vi "MegaAwesome_8_29_12d_JW.vi"() -> ()   [LabVIEW 2011]
uses:
  MegaAwesome_States.ctl
  <vilib>/Utility/file.llb/Read From Spreadsheet File (string).vi
  <vilib>/Utility/file.llb/Write To Spreadsheet File (string).vi
panel:
  out "Opj X Axis":string
  out "X Axis Display Type":string
  in  "Index-Sat":dbl=5.0
  in  "Index-Lin":dbl=5.0
  in  "IndexLog-Lin":dbl=5.0
  in  "IndexLog-Sat":dbl=5.0 caption="Num Pts"
  out "Lin Id-Log Used":dbl[](array[numeric])
  out "Lin-Vg Array-Log Used":dbl[](array[numeric])
  out "Total Width":dbl
  in  "New: Comments":string
  out "Save Array":string[][](array[string])
  out "Folder Index":i32 caption="Length"
  out "Sat Id-Used":dbl[](array[numeric])
  out "Sat Vg Array-Used":dbl[](array[numeric])
  out "Vg Array-Log-Used":dbl[](array[numeric])
  out "Sat Id-Log-Used":dbl[](array[numeric])
  out "Lin Id-Used":dbl[](array[numeric])
  out "Lin-Vg Array-Used":dbl[](array[numeric])
  out "Lin Vd":dbl
  out "Recorded Prop":T1
  out "Current State":T2
  in  "Main Tab Control":T3(tab)
  in  "Image Folder":path
  out "Image File":path=path "D:/UserData/Desktop/Jeremy/WFU/Research/Programs/VI mods/Image Not Found.png"
  in  "Transfer File":path
  out "Transfer Folder":path
  out "Fabrication Prop":T4
  in  "Transfer Plots":T5(tab)=enum."Saturation"
  in  "Lin-Trans Slider":dbl(slide) step=1.0 scale=-22.0..89.0 scale format="%#_1p"
  out "Sqrt-Lin":cluster{dbl[], dbl[]}[](graph)
  in  "Next Sqrt Lin":bool
  in  "Previous Sqrt Lin":bool
  in  "Sat-Trans Slider":dbl(slide) step=1.0 scale=-40.0..40.0 scale format="%#_1p"
  out "Sqrt-Sat":cluster{dbl[], dbl[]}[](graph)
  in  "Previous Sqrt Sat":bool
  in  "Next Sqrt Sat":bool
  out "Raw- Lin":cluster{dbl[], dbl[]}[](graph)
  out "Raw- Sat":cluster{dbl[], dbl[]}[](graph)
  in  "Log Plots":enum32{"Linear", "Saturation", "Transport"}(tab)=enum."Saturation"
  in  "Lin-Log Slider":dbl(slide) step=1.0 scale=-1.0..82.0 scale format="%#_1p"
  in  "Previous Log Lin":bool
  in  "Next Log Lin":bool
  out "Log-Lin":cluster{dbl[], dbl[]}[](graph)
  in  "Sat-Log Slider":dbl(slide) step=1.0 scale=-1.0..82.0 scale format="%#_1p"
  in  "Previous Log Sat":bool
  in  "Next Log Sat":bool
  out "Sat-Log":cluster{dbl[], dbl[]}[](graph)
  out "Transport":cluster{dbl[], dbl[]}[](graph)
  in  "Manual Controls":T6
  in  "File Controls":T7
  out "Date Recorded":string="Date Recorded" caption="Measured"
  out "Data Name:":string
  out "Image Name":string
  out "Index":string
  out "Date Created":string caption="Fabricated"
  in  "Comments:":string
  out "Rec: Length":dbl caption="Length" format="%#_3g"
  out "Rec: Width":dbl caption="Width" format="%#_4g"
  out "Rec: Dielectric (d)":dbl caption="Dielectric (d)" format="%#_3g"
  in  "New: Dielectric":dbl
  in  "New: Length":dbl
  in  "New: Width":dbl
  out "Rec: Temp":dbl caption="Sample Temp" format="%.1f"
  in  "New: Temp":dbl format="%.1f"
  out "Image Out":T8(plugin-control)
  in  "Num Pts":dbl=5.0
  in  "Num Pts Log":dbl=5.0 caption="Num Pts"
  out "Recorded Values Cluster":T9
  out "Calculated Values Cluster":T9 caption="Recorded Values Cluster"
  out "Re-Calculated Values Cluster":T9 caption="Recorded Values Cluster"
  in  "Independant Variable:":string(combo)="Length (um):"
  out "Image Preview":T8(plugin-control)
  in  "No Image File":path=path "\\\\acad1\\physics/Jurchescu-group/JW-PD/Mega Awesome/Image Not Found.png"
  in  "Room Temp":dbl=294.0
  in  "Origin Project File":path=path "\\\\acad1\\physics/Jurchescu-group/JW-PD/Group Library/Origin Project Files/DeviceData_8_10_12a_JW.opj"
  # "Image Location"
  # "Recorded"
  # "Calculated"
  # "Re-Calculated"
  # "Manual"
  # "Used points display at y=0"
  # "Slider\nDoesn't\nWork"
  # "Slider\nDoesn't\nWork"
  # "No new points displayed"
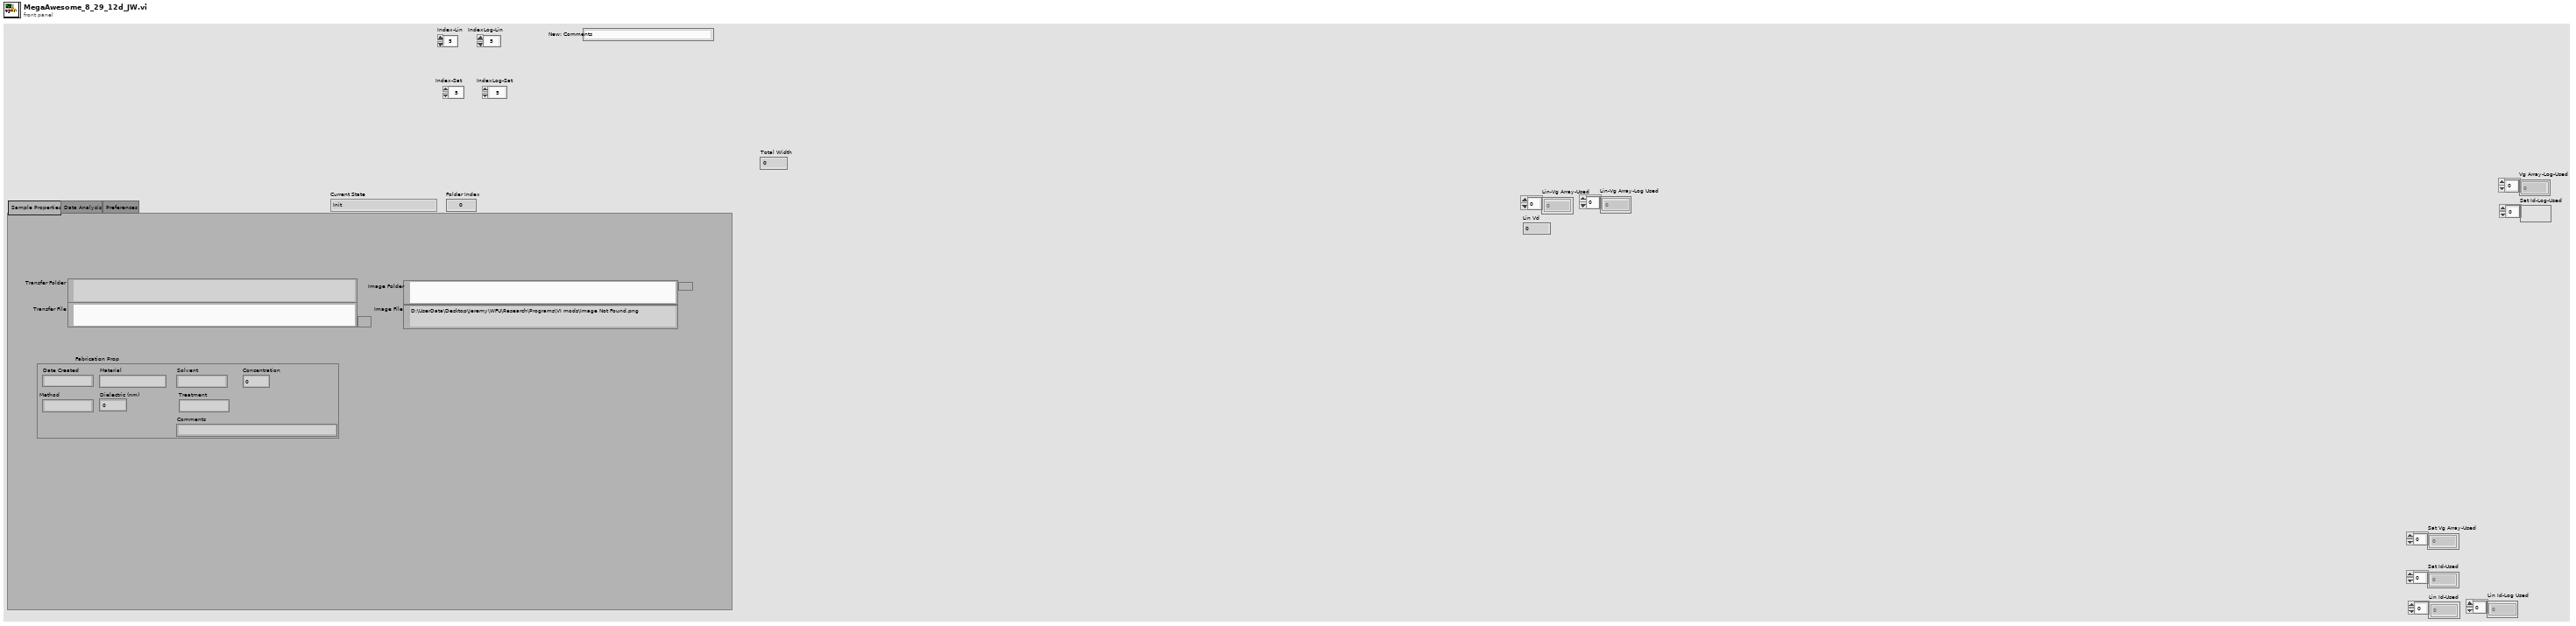
[diagram p1: front panel]
types:
  T1 = cluster{"Date Recorded":string, "Index":string, "Length":dbl, "Width":dbl, "Sample Temp":dbl}
  T2 = typedef "MegaAwesome_States.ctl" = enum16{"Init", "File Missing", "No Event", "Read Data", "Calculated Values", "Re-Calculated Values", "Next File", "Previous File", "Discard File", "Save", "Save Lines", "Export", "Exit"}
  T3 = enum32{"Sample Properties", "Data Analysis", "Preferences"}
  T4 = cluster{"Date Created":string, "Material":string, "Solvent":string, "Concentration":dbl, "Method":string, "Dielectric (nm)":dbl, "Treatment":string, "Comments":string}
  T5 = enum32{"Linear", "Saturation", "Raw-Linear", "Raw-Saturation"}
  T6 = cluster{"Manual-Temp":bool, "Manual-Width":bool, "Manuel-Length":bool, "Manuel-Dielectric":bool, "Manual Comments":bool}
  T7 = cluster{"Previous File":bool, "Discard ":bool, "Save Lines":bool, "Close":bool, "Next File ":bool, "Save":bool, "Save Next":bool, "Export":bool}
  T8 = typedef "IMAQ Image.ctl" = refnum<image>
  T9 = cluster{"Mobility-Sat":dbl, "Moblitity-Lin":dbl, "On/Off":dbl, "Off Current":dbl, "Vt-Sat":dbl, "STS":dbl, "Trap Density-VT":dbl, "Trap Density-STS":dbl}
  T10 = cluster{"[0]":cluster{dbl[], dbl[]}, "[1]":cluster{dbl[], dbl[]}, "[2]":cluster{dbl[], dbl[]}, "[3]":cluster{dbl[], dbl[]}, "[4]":cluster{dbl[], dbl[]}, "[5]":cluster{dbl[], dbl[]}, "[6]":cluster{dbl[], dbl[]}, "[7]":cluster{dbl[], dbl[]}, "[8]":cluster{dbl[], dbl[]}}
  T11 = cluster{"Sat Vg Used":dbl[], "Sat Sqrt(Id) Used ":dbl[], "Lin Vg Used":dbl[], "Lin Sqrt(Id) Used":dbl[], "Index-Lin":dbl, "Index-Sat":dbl}
  T12 = cluster{"Raw Sat":cluster{dbl[], dbl[]}[], "Sqrt Sat":cluster{dbl[], dbl[]}[], "Log Sat":cluster{dbl[], dbl[]}[], "Raw Lin":cluster{dbl[], dbl[]}[], "Sqrt Lin":cluster{dbl[], dbl[]}[], "Log Lin":cluster{dbl[], dbl[]}[]}
  T13 = cluster{"Mobility-Sat":dbl, "Vt-Sat":dbl, "Mobility-Lin":dbl, "Vt-Lin":dbl, "Off I-Sat":dbl, "On/Off I-Sat":dbl}
  T14 = cluster{"Sat Vg Used":dbl[], "Sat Log(Id) Used":dbl[], "Lin Vg Used":dbl[], "Lin Log(Id) Used":dbl[], "STS Index-Sat":dbl, "STS Index-Lin":dbl}
  T15 = cluster{"Independant  Variable Indicator":string, "Parameter String Indicator":string}
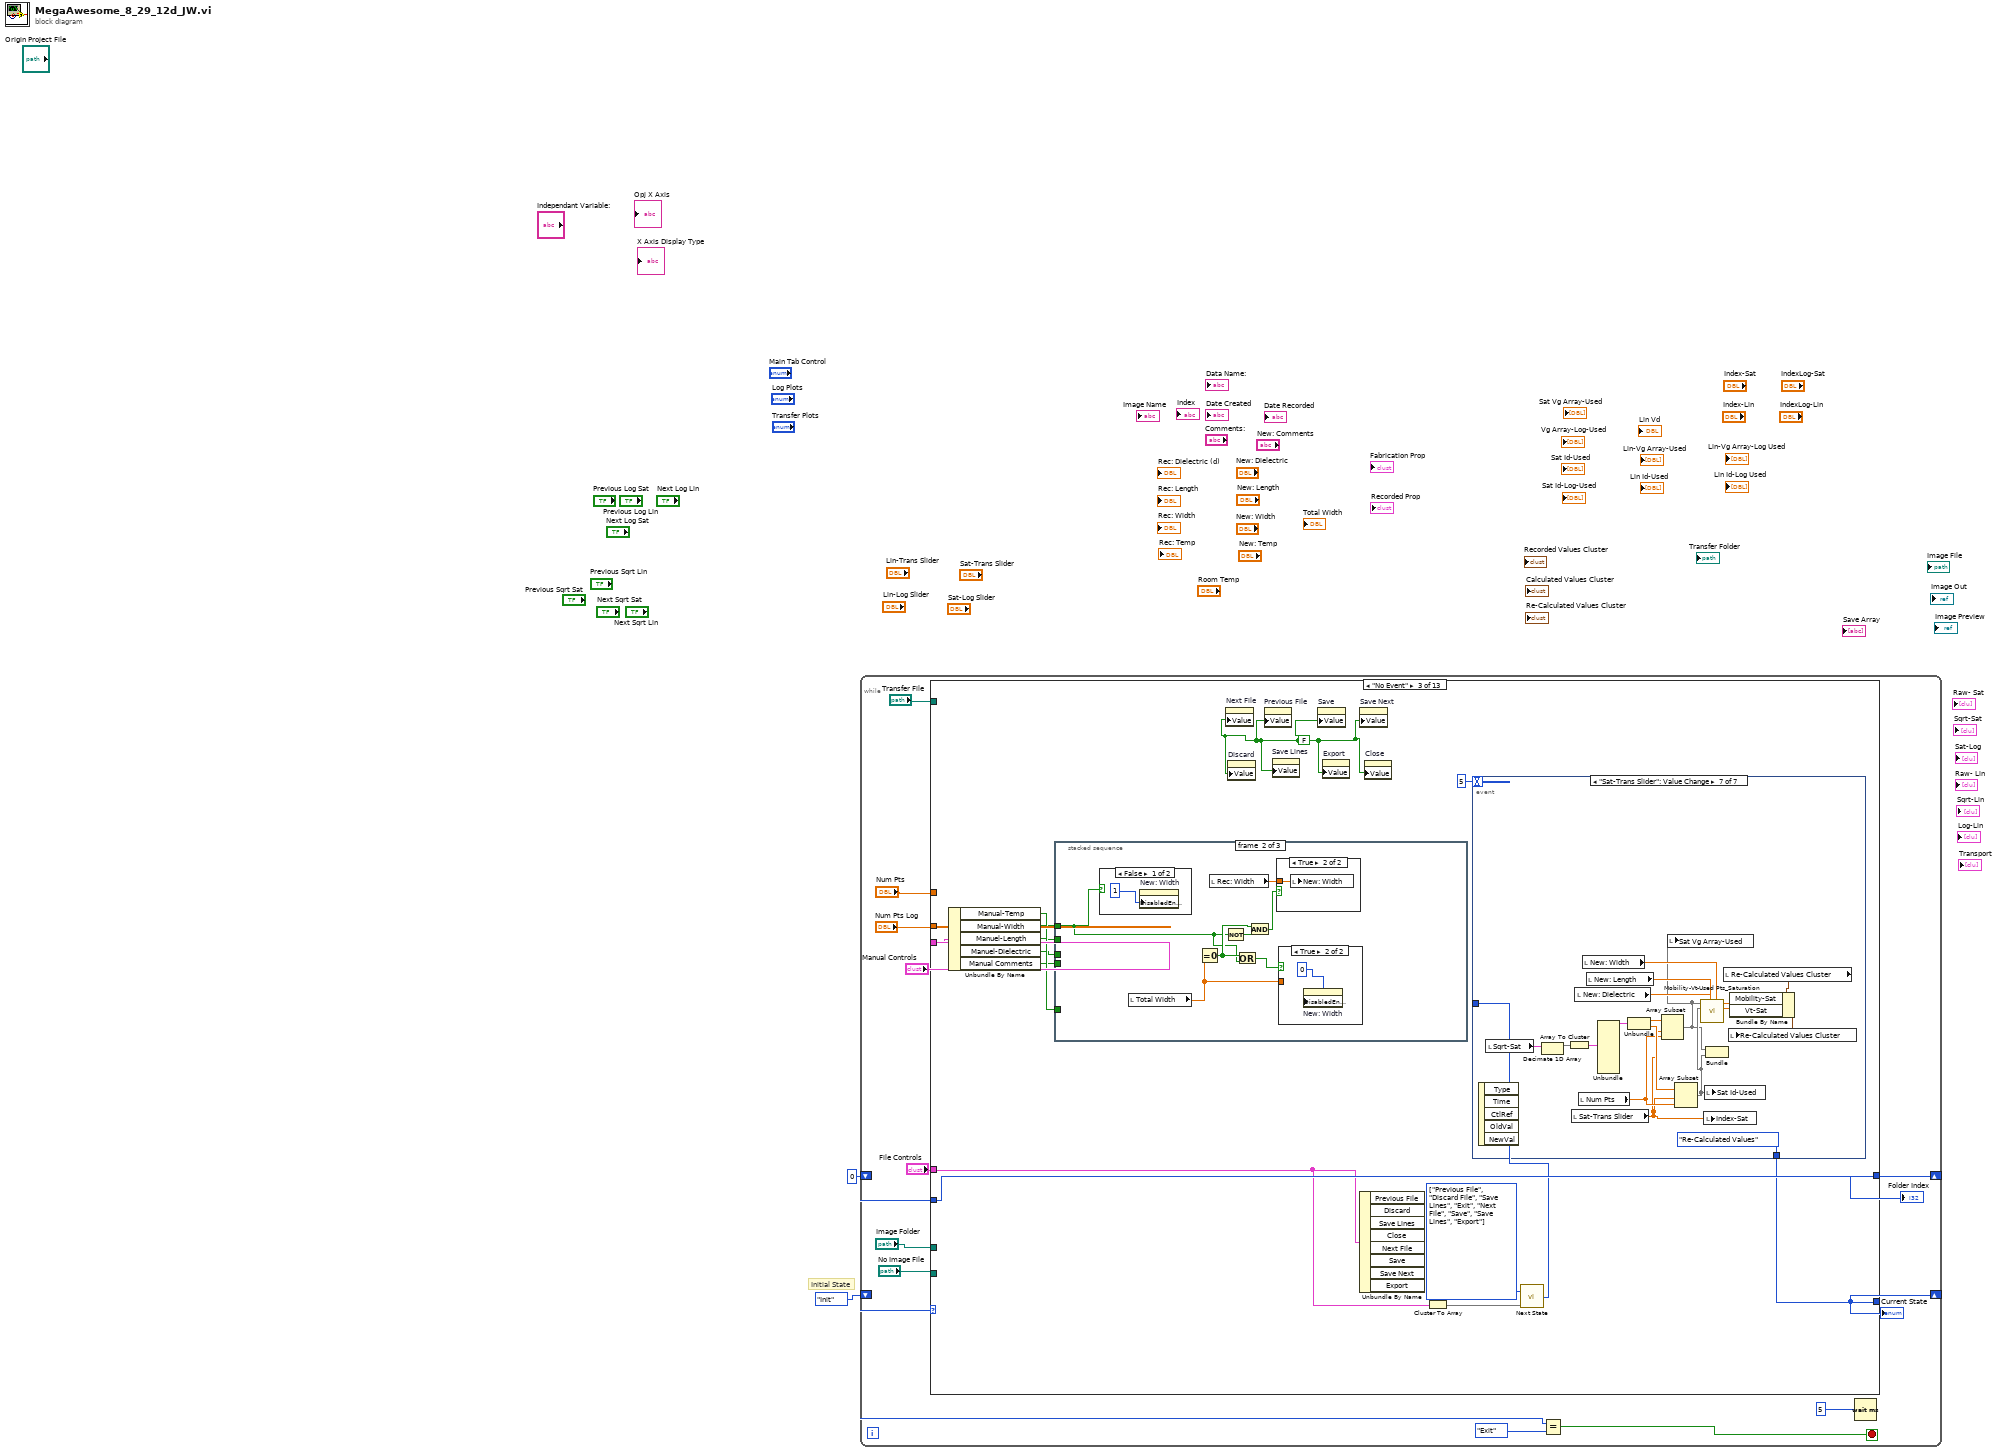
[diagram p0: block diagram]
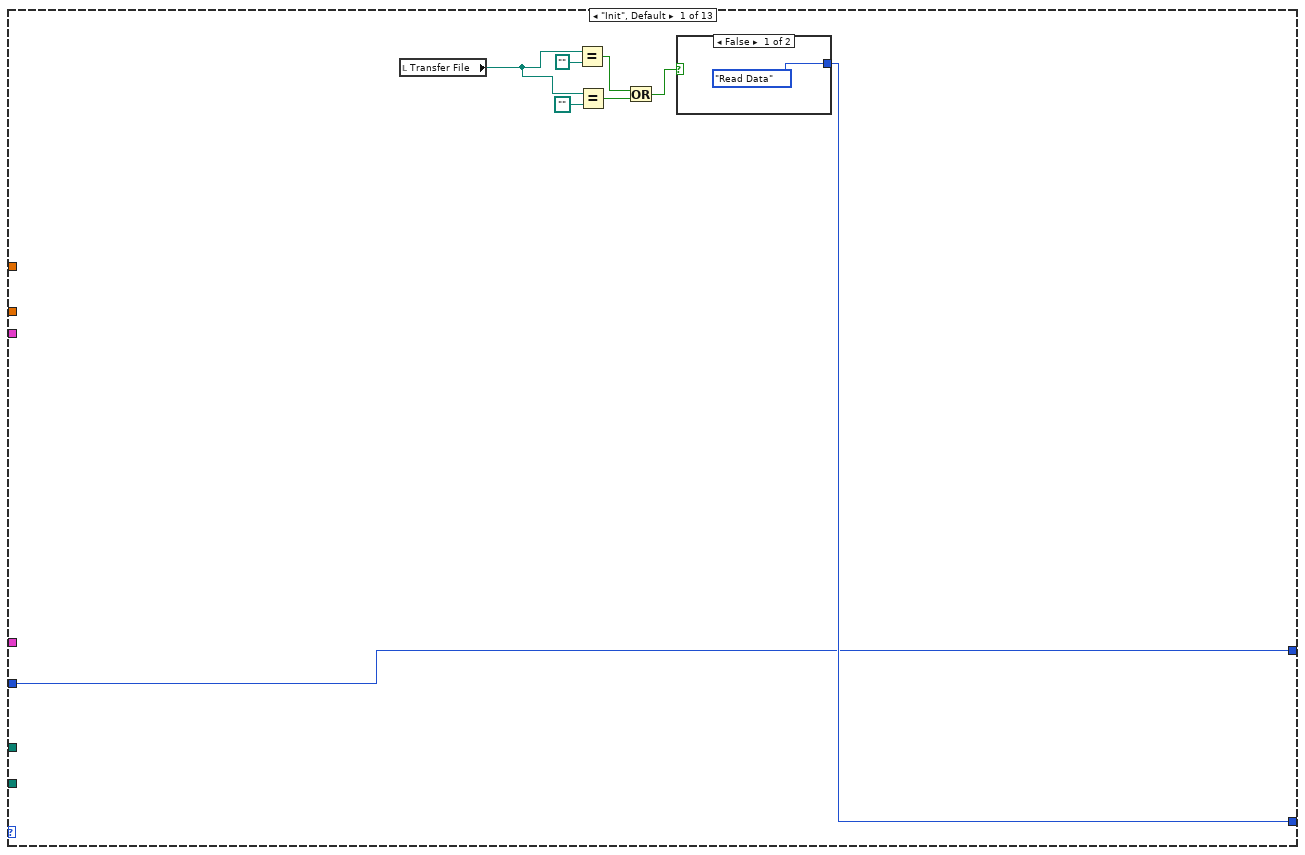
[diagram p2: hidden frame]
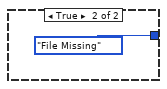
[diagram p3: hidden frame]
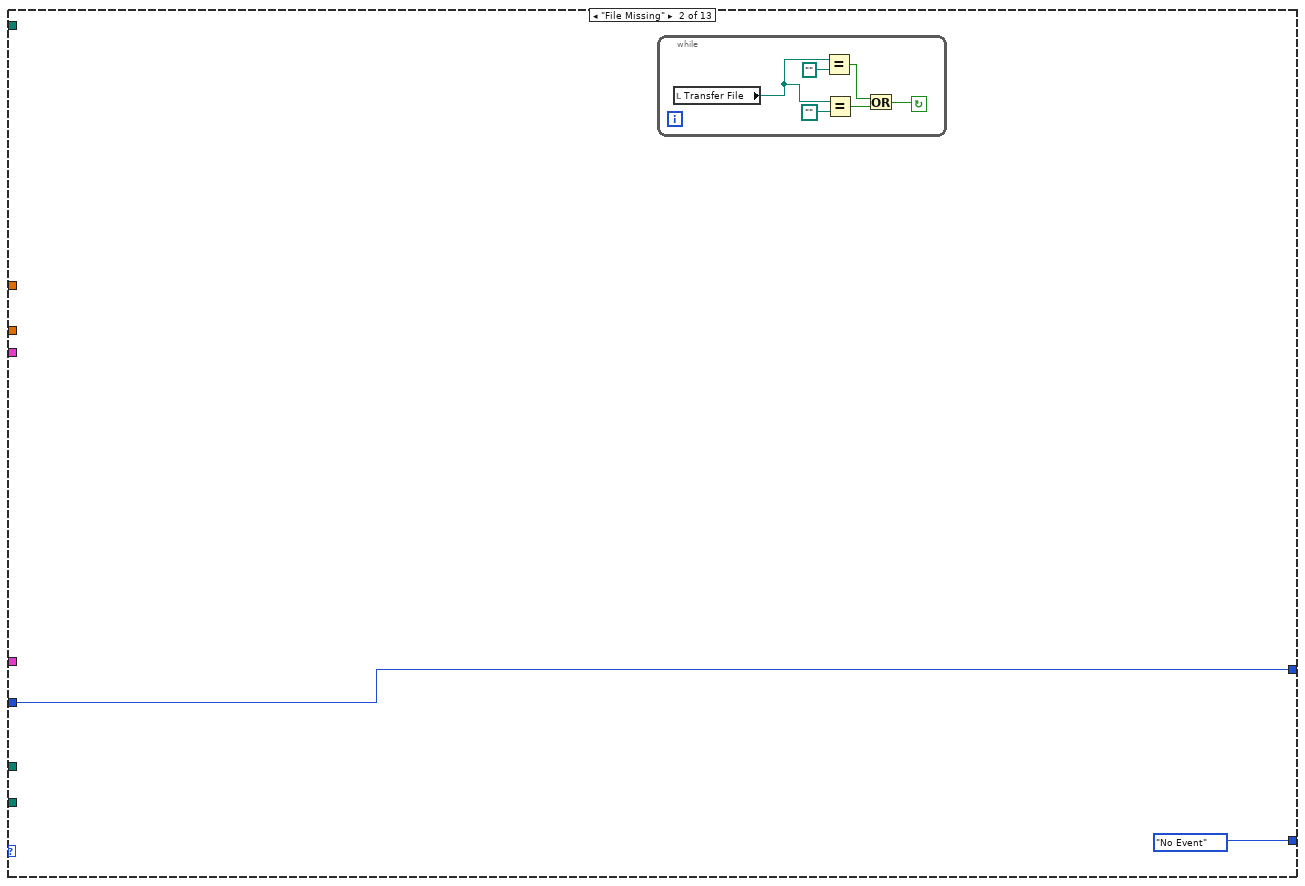
[diagram p4: hidden frame]
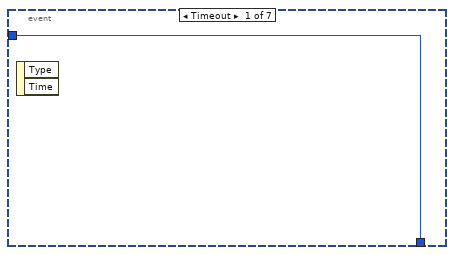
[diagram p5: hidden frame]
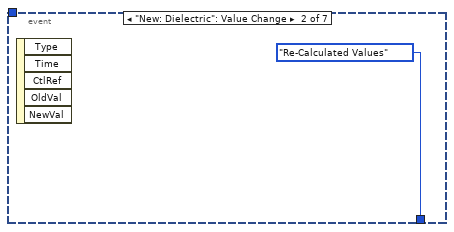
[diagram p6: hidden frame]
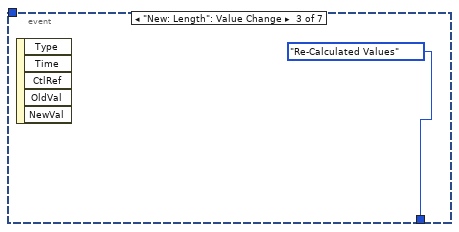
[diagram p7: hidden frame]
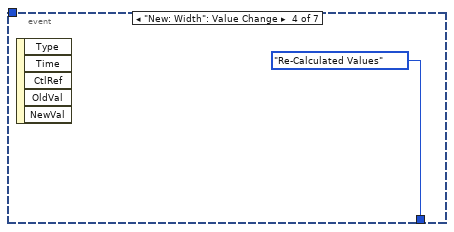
[diagram p8: hidden frame]
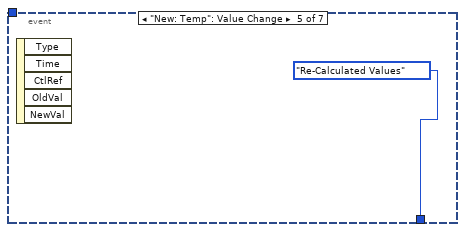
[diagram p9: hidden frame]
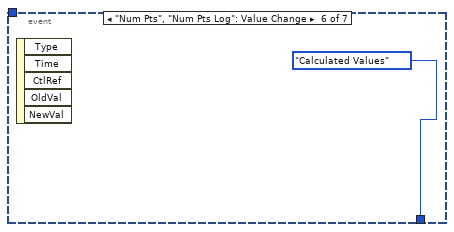
[diagram p10: hidden frame]
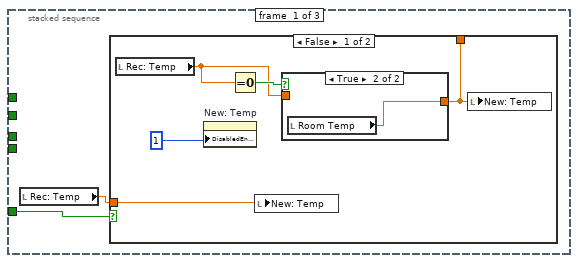
[diagram p11: hidden frame]
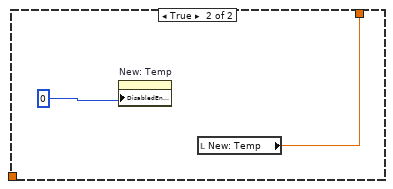
[diagram p13: hidden frame]
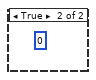
[diagram p14: hidden frame]
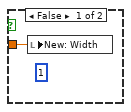
[diagram p16: hidden frame]
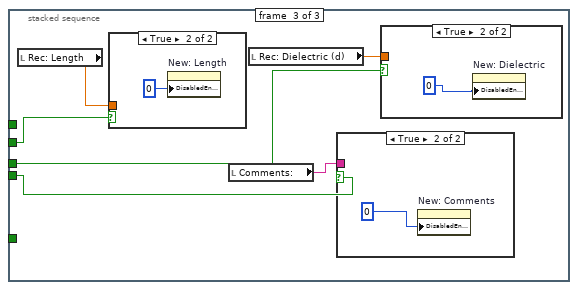
[diagram p17: hidden frame]
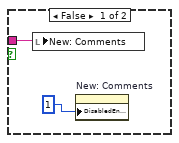
[diagram p18: hidden frame]
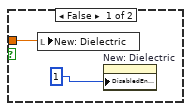
[diagram p19: hidden frame]
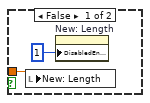
[diagram p20: hidden frame]
diagram:
  # "Initial State"
  n1 = while {
    shift-right: [w13] -> _
    shift-left: MegaAwesome_States."Init" -> [w15]
    shift-right: [w6] -> _
    shift-left: 0 -> [w7]
    stop <- w16 stop-if-true
    n2 = case shown="\"No Event\"" w15 {
      tunnel: [w18 MegaAwesome_States."No Event" w37 MegaAwesome_States."Calculated Values" MegaAwesome_States."Re-Calculated Values" MegaAwesome_States."No Event" MegaAwesome_States."Read Data" MegaAwesome_States."Read Data" MegaAwesome_States."No Event" w261 MegaAwesome_States."No Event" MegaAwesome_States."No Event" MegaAwesome_States."Exit"] -> w13
      tunnel: "Transfer File" -> [_ _ _ w116 w162 _ w230 w242 _ w266 _ _ _]
      tunnel: "Num Pts" -> [_ _ _ _ w166 _ _ _ _ _ _ _ _]
      tunnel: "Num Pts Log" -> [_ _ _ _ w165 _ _ _ _ _ _ _ _]
      tunnel: "Image Folder" -> [_ _ _ _ w161 _ _ _ _ _ _ _ _]
      tunnel: "No Image File" -> [_ _ _ _ w160 _ _ _ _ _ _ _ _]
      tunnel: [w17 w27 w45 w110 w159 w190 w215 w240 w258 w267 w782 w785 w786] -> w6
      tunnel: w7 -> [w17 w27 w45 _ w159 w190 w216 w241 w258 w267 w782 w785 w786]
      tunnel: "Manual Controls" -> [_ _ w39 _ _ _ _ _ _ w265 _ _ _]
      tunnel: "File Controls" -> [_ _ w35 _ _ _ _ _ _ w260 _ _ _]
      frame "Init", Default {
        n3 = local read "Transfer File"() -> (w19:path)
        n4 = Equal?(x=w19, y=path "") -> (x = y?=w22:bool)
        n5 = Equal?(x=w19, y=path "") -> (x = y?=w21:bool)
        n6 = Or(x=w22, y=w21) -> (x .or. y?=w24:bool)
        n7 = case shown="False" w24 {
          tunnel: [MegaAwesome_States."Read Data" MegaAwesome_States."File Missing"] -> w18
          frame False {
          }
          frame True {
          }
        }
      }
      frame "File Missing" {
        n8 = while {
          stop <- w29 continue-if-true
          n9 = local read "Transfer File"() -> (w30:path)
          n10 = Equal?(x=w30, y=path "") -> (x = y?=w32:bool)
          n11 = Equal?(x=w30, y=path "") -> (x = y?=w33:bool)
          n12 = Or(x=w32, y=w33) -> (x .or. y?=w29:bool)
        }
      }
      frame "No Event" {
        w47 = T2[] [enum."Previous File", enum."Discard File", enum."Save Lines", enum."Exit", enum."Next File", enum."Save", enum."Save Lines", enum."Export"] items=["Init", "File Missing", "No Event", "Read Data", "Calculated Values", "Re-Calculated Values", "Next File", "Previous File", "Discard File", "Save", "Save Lines", "Export", "Exit"]
        w48 = FALSE
        n13 = Unbundle By Name(w39) -> ("Manual-Temp"=w44:bool, "Manual-Width"=w43:bool, "Manuel-Length"=w42:bool, "Manuel-Dielectric"=w41:bool, "Manual Comments"=w40:bool)
        n14 = stacked-sequence {
          tunnel: w44 -> [w74 _ _]
          tunnel: w43 -> [_ w84 _]
          tunnel: w42 -> [_ _ w99]
          tunnel: w41 -> [_ _ w96]
          tunnel: w40 -> [_ _ w95]
          frame #0 {
            n15 = local read "Rec: Temp"() -> (w73:dbl)
            n16 = case shown="False" w74 {
              tunnel: w73 -> [w79 _]
              tunnel: [w76 w83] -> _
              frame False {
                n17 = local read "Rec: Temp"() -> (w77:dbl)
                n18 = property on="New: Temp" class="DigNum (strict)"("DisabledEnum"=1) -> ()  [unwired: 2 in, 2 out]
                n19 = Equal To 0?(x=w77) -> (x = 0?=w78:bool)
                n20 = local write "New: Temp"(w79) -> ()
                n21 = case shown="True" w78 {
                  tunnel: [w80 w81] -> w76
                  tunnel: w77 -> [w80 _]
                  frame False {
                  }
                  frame True {
                    n22 = local read "Room Temp"() -> (w81:dbl)
                  }
                }
                n23 = local write "New: Temp"(w76) -> ()
              }
              frame True {
                n24 = property on="New: Temp" class="DigNum (strict)"("DisabledEnum"=0) -> ()  [unwired: 2 in, 2 out]
                n25 = local read "New: Temp"() -> (w83:dbl)
              }
            }
          }
          frame #1 {
            n26 = case shown="False" w84 {
              frame False {
                n27 = property on="New: Width" class="DigNum (strict)"("DisabledEnum"=1) -> ()  [unwired: 2 in, 2 out]
              }
              frame True {
                (unwired) 0
              }
            }
            n28 = local read "Total Width"() -> (w90:dbl)
            n29 = Equal To 0?(x=w90) -> (x = 0?=w87:bool)
            n30 = local read "Rec: Width"() -> (w88:dbl)
            n31 = Not(x=w84) -> (.not. x?=w86:bool)
            n32 = Or(x=w87, y=w84) -> (x .or. y?=w89:bool)
            n33 = And(x=w87, y=w86) -> (x .and. y?=w85:bool)
            n34 = case shown="True" w85 {
              tunnel: w88 -> [_ w92]
              frame False {
              }
              frame True {
                n35 = local write "New: Width"(w92) -> ()
              }
            }
            n36 = case shown="True" w89 {
              tunnel: w90 -> [w93 _]
              frame False {
                (unwired) 1
                n37 = local write "New: Width"(w93) -> ()
              }
              frame True {
                n38 = property on="New: Width" class="DigNum (strict)"("DisabledEnum"=0) -> ()  [unwired: 2 in, 2 out]
              }
            }
          }
          frame #2 {
            n39 = local read "Rec: Length"() -> (w100:dbl)
            n40 = case shown="True" w99 {
              tunnel: w100 -> [w108 _]
              frame False {
                n41 = local write "New: Length"(w108) -> ()
                n42 = property on="New: Length" class="DigNum (strict)"("DisabledEnum"=1) -> ()  [unwired: 2 in, 2 out]
              }
              frame True {
                n43 = property on="New: Length" class="DigNum (strict)"("DisabledEnum"=0) -> ()  [unwired: 2 in, 2 out]
              }
            }
            n44 = local read "Comments:"() -> (w97:string)
            n45 = local read "Rec: Dielectric (d)"() -> (w98:dbl)
            n46 = case shown="True" w95 {
              tunnel: w97 -> [w102 _]
              frame False {
                n47 = local write "New: Comments"(w102) -> ()
                n48 = property on="New: Comments" class="Str"("DisabledEnum"=1) -> ()  [unwired: 2 in, 2 out]
              }
              frame True {
                n49 = property on="New: Comments" class="Str"("DisabledEnum"=0) -> ()  [unwired: 2 in, 2 out]
              }
            }
            n50 = case shown="True" w96 {
              tunnel: w98 -> [w105 _]
              frame False {
                n51 = local write "New: Dielectric"(w105) -> ()
                n52 = property on="New: Dielectric" class="DigNum (strict)"("DisabledEnum"=1) -> ()  [unwired: 2 in, 2 out]
              }
              frame True {
                n53 = property on="New: Dielectric" class="DigNum (strict)"("DisabledEnum"=0) -> ()  [unwired: 2 in, 2 out]
              }
            }
          }
        }
        n54 = property on="Next File" class="Bool (strict)"("Value"=w48) -> ()  [unwired: 2 in, 2 out]
        n55 = property on="Discard" class="Bool (strict)"("Value"=w48) -> ()  [unwired: 2 in, 2 out]
        n56 = property on="Previous File" class="Bool (strict)"("Value"=w48) -> ()  [unwired: 2 in, 2 out]
        n57 = property on="Save Lines" class="Bool (strict)"("Value"=w48) -> ()  [unwired: 2 in, 2 out]
        n58 = property on="Save" class="Bool (strict)"("Value"=w48) -> ()  [unwired: 2 in, 2 out]
        n59 = property on="Export" class="Bool (strict)"("Value"=w48) -> ()  [unwired: 2 in, 2 out]
        n60 = Unbundle By Name(w35) -> ()  [unwired: 8 out]
        n61 = property on="Save Next" class="Bool (strict)"("Value"=w48) -> ()  [unwired: 2 in, 2 out]
        n62 = property on="Close" class="Bool (strict)"("Value"=w48) -> ()  [unwired: 2 in, 2 out]
        n63 = Cluster To Array(cluster=w35) -> (array=w46:bool[])
        n64 = call "Next State.vi"("Buttons []"=w46, "States []"=w47) -> ("Enum"=w38:T2)
        n65 = event shown="[6] \"Sat-Trans Slider\": Value Change" {
          selector: _ -> [_ _ _ _ _ _ _]
          dyn-events: _ -> [_ _ _ _ _ _ _]
          timeout: 5 -> [_ _ _ _ _ _ _]
          tunnel: w38 -> [w49 _ _ _ _ _ _]
          tunnel: [w49 MegaAwesome_States."Re-Calculated Values" MegaAwesome_States."Re-Calculated Values" MegaAwesome_States."Re-Calculated Values" MegaAwesome_States."Re-Calculated Values" MegaAwesome_States."Calculated Values" MegaAwesome_States."Re-Calculated Values"] -> w37
          event Timeout {
            n66 = event-data() -> ()  [unwired: 1 in, 2 out]
          }
          event "New: Dielectric": Value Change {
            n67 = event-data() -> ()  [unwired: 1 in, 5 out]
          }
          event "New: Length": Value Change {
            n68 = event-data() -> ()  [unwired: 1 in, 5 out]
          }
          event "New: Width": Value Change {
            n69 = event-data() -> ()  [unwired: 1 in, 5 out]
          }
          event "New: Temp": Value Change {
            n70 = event-data() -> ()  [unwired: 1 in, 5 out]
          }
          event "Num Pts", "Num Pts Log": Value Change {
            n71 = event-data() -> ()  [unwired: 1 in, 5 out]
          }
          event "Sat-Trans Slider": Value Change {
            n72 = event-data() -> ()  [unwired: 1 in, 5 out]
            n73 = local read "Sqrt-Sat"() -> (w72:cluster{dbl[], dbl[]}[])
            n74 = Decimate 1D Array(w72) -> (w71:cluster{dbl[], dbl[]}[])  [unwired: 1 out]
            n75 = Array To Cluster(array=w71) -> (cluster=w70:T10)
            n76 = local read "Sat-Trans Slider"() -> (w65:dbl)
            n77 = local read "New: Dielectric"() -> (w62:dbl)
            n78 = local read "Num Pts"() -> (w66:dbl)
            n79 = local read "New: Width"() -> (w64:dbl)
            n80 = local read "New: Length"() -> (w63:dbl)
            n81 = Unbundle(w70) -> ("[0]"=w69:cluster{dbl[], dbl[]})  [unwired: 8 out]
            n82 = Unbundle(w69) -> (w68:dbl[], w67:dbl[])
            n83 = Array Subset(array=w68, index=w65, length=w66) -> (w60:dbl[])
            n84 = local write "Sat Vg Array-Used"(w60) -> ()
            n85 = Array Subset(array=w67, index=w65, length=w66) -> (w61:dbl[])
            n86 = call "Mobility-Vt-Used Pts_Saturation.vi"("Width"=w64, "Length"=w63, "Dielectric (d)"=w62, "Sat Id Used"=w61, "Vg Used"=w60) -> ("Vt"=w56:dbl, "Mobility"=w57:dbl)  [unwired: 4 in, 1 out]
            n87 = local write "Index-Sat"(w65) -> ()
            n88 = local write "Sat Id-Used"(w61) -> ()
            n89 = Bundle(w60, w61) -> ()  [unwired: 1 in, 1 out]
            n90 = local read "Re-Calculated Values Cluster"() -> (w59:T9)
            n91 = Bundle By Name(cluster=w59, "Mobility-Sat"=w57, "Vt-Sat"=w56) -> (w58:T9)
            n92 = local write "Re-Calculated Values Cluster"(w58) -> ()
          }
        }
      }
      frame "Read Data" {
        n93 = call "Recorded Values.vi"("Path"=w116) -> ("Recorded Char"=w134:T9, "Recorded Prop"=w124:T1, "Fabrication Prop"=w118:T4)  [unwired: 8 in]
        n94 = Strip Path(path=w116) -> (stripped path=w117:path, name=w115:string)
        n95 = local write "Fabrication Prop"(w118) -> ()
        n96 = local write "Recorded Prop"(w124) -> ()
        n97 = Unbundle By Name(w124) -> ("Date Recorded"=w123:string, "Index"=w121:string, "Length"=w122:dbl, "Width"=w120:dbl, "Sample Temp"=w119:dbl)
        n98 = local write "Recorded Values Cluster"(w134) -> ()
        n99 = Unbundle By Name(w124) -> ("Sample Temp"=w127:dbl)
        n100 = Unbundle By Name(w118) -> ("Dielectric (nm)"=w112:dbl, "Comments"=w111:string)
        n101 = List Folder(path=w117) -> (filenames=w113:string[])  [unwired: 3 in, 3 out]
        n102 = local write "Rec: Dielectric (d)"(w112) -> ()
        n103 = local write "Date Created"(w123) -> ()
        n104 = local write "Index"(w121) -> ()
        n105 = local write "Rec: Length"(w122) -> ()
        n106 = local write "Rec: Width"(w120) -> ()
        n107 = local write "Rec: Temp"(w119) -> ()
        n108 = Equal To 0?(x=w127) -> (x = 0?=w130:bool)
        n109 = Number To Decimal String(number=w127) -> (decimal integer string=w131:string)  [unwired: 1 in]
        n110 = local write "Comments:"(w111) -> ()
        n111 = Search 1D Array(1D array=w113, element=w115) -> (index of element=w110:i32)  [unwired: 1 in]
        n112 = Equal?(x="", y=w131) -> (x = y?=w129:bool)
        n113 = Index Array(array=w113, index=w110) -> (element=w114:string)
        n114 = Or(x=w130, y=w129) -> (x .or. y?=w128:bool)
        n115 = local write "Data Name:"(w114) -> ()
        n116 = case shown="False" w128 {
          tunnel: [w135 w136] -> w125
          tunnel: w127 -> [w135 _]
          frame False {
          }
          frame True {
            n117 = local read "Room Temp"() -> (w136:dbl)
          }
        }
        n118 = local write "New: Temp"(w125) -> ()
        n119 = Bundle By Name(cluster=w124, "Sample Temp"=w125) -> (w126:T1)
        n120 = local write "Recorded Prop"(w126) -> ()
      }
      frame "Calculated Values" {
        n121 = local read "Fabrication Prop"() -> (w171:T4)
        n122 = local read "Recorded Prop"() -> (w164:T1)
        n123 = disable-structure shown="Disabled" {
          disable-tunnel: w162 -> [w188 _]
          disable-tunnel: w161 -> [w187 _]
          disable-tunnel: w160 -> [w186 _]
          frame Disabled {
            n124 = call "Image from TRF Display.vi"("No Image File"=w186, "Image Folder"=w187, "Transfer File"=w188) -> ("Image Out 2"=w182:T8, "Image Out"=w183:T8, "Image File"=w184:path, "Image Name"=w185:string)  [unwired: 5 in]
            n125 = local write "Image File"(w184) -> ()
            n126 = local write "Image Name"(w185) -> ()
            n127 = local write "Image Out"(w183) -> ()
            n128 = local write "Image Preview"(w182) -> ()
          }
          frame Enabled {
          }
        }
        n129 = local read "Calculated Values Cluster"() -> (w181:T9)
        n130 = call "Mobility-Vt Calculator-File.vi"("NumPts"=w166, "Path"=w162) -> ("Used Points"=w158:T11, "Graph Cluster"=w145:T12, "Lin Vd"=w154:dbl, "Output"=w179:T13)  [unwired: 6 in]
        n131 = call "STS Calculator-File.vi"("NumPts"=w165, "Path"=w162) -> ("Used Points"=w152:T14, "Ouput"=w174:cluster{"STS-Sat":dbl, "STS-Lin":dbl})  [unwired: 6 in, 2 out]
        n132 = Unbundle By Name(w171) -> ("Dielectric (nm)"=w169:dbl)
        n133 = Unbundle By Name(w164) -> ("Sample Temp"=w163:dbl)
        n134 = Unbundle By Name(w179) -> ("Mobility-Sat"=w178:dbl, "Vt-Sat"=w170:dbl, "Mobility-Lin"=w177:dbl, "Off I-Sat"=w176:dbl, "On/Off I-Sat"=w175:dbl)  [unwired: 1 out]
        n135 = local write "Lin Vd"(w154) -> ()
        n136 = Unbundle By Name(w174) -> ("STS-Sat"=w168:dbl)  [unwired: 1 out]
        n137 = call "Trap Density_VT.vi"("VT"=w170, "Dielectric"=w169) -> ("Trap Density-VT"=w173:dbl)
        n138 = call "Trap Density_STS.vi"("Temp (T) [K]"=w163, "S.T.S. (S)"=w168, "Dielectric"=w169) -> ("Trap Density (N)"=w172:dbl)  [unwired: 8 in]
        n139 = Bundle By Name(cluster=w181, "Mobility-Sat"=w178, "Moblitity-Lin"=w177, "On/Off"=w175, "Off Current"=w176, "Vt-Sat"=w170, "STS"=w168, "Trap Density-VT"=w173, "Trap Density-STS"=w172) -> (w180:T9)
        n140 = Unbundle By Name(w158) -> ("Sat Vg Used"=w157:dbl[], "Sat Sqrt(Id) Used"=w156:dbl[], "Lin Vg Used"=w155:dbl[], "Lin Sqrt(Id) Used"=w153:dbl[], "Index-Lin"=w138:dbl, "Index-Sat"=w137:dbl)
        n141 = Unbundle By Name(w152) -> ("Sat Vg Used"=w149:dbl[], "Sat Log(Id) Used"=w148:dbl[], "Lin Vg Used"=w147:dbl[], "Lin Log(Id) Used"=w146:dbl[], "STS Index-Sat"=w151:dbl, "STS Index-Lin"=w150:dbl)
        n142 = local write "Calculated Values Cluster"(w180) -> ()
        n143 = local write "Vg Array-Log-Used"(w149) -> ()
        n144 = local write "Sat Id-Log-Used"(w148) -> ()
        n145 = local write "Lin-Vg Array-Log Used"(w147) -> ()
        n146 = local write "Lin Id-Log Used"(w146) -> ()
        n147 = local write "IndexLog-Sat"(w151) -> ()
        n148 = local write "Index-Lin"(w150) -> ()
        n149 = local write "Sat Vg Array-Used"(w157) -> ()
        n150 = local write "Sat Id-Used"(w156) -> ()
        n151 = local write "Lin-Vg Array-Used"(w155) -> ()
        n152 = local write "Lin Id-Used"(w153) -> ()
        n153 = local write "Index-Sat"(w137) -> ()
        n154 = local write "Index-Lin"(w138) -> ()
        n155 = local write "Sat-Trans Slider"(w137) -> ()
        n156 = local write "Lin-Trans Slider"(w138) -> ()
        n157 = Unbundle By Name(w145) -> ("Raw Sat"=w140:cluster{dbl[], dbl[]}[], "Sqrt Sat"=w139:cluster{dbl[], dbl[]}[], "Log Sat"=w144:cluster{dbl[], dbl[]}[], "Raw Lin"=w143:cluster{dbl[], dbl[]}[], "Sqrt Lin"=w142:cluster{dbl[], dbl[]}[], "Log Lin"=w141:cluster{dbl[], dbl[]}[])
        n158 = local write "Raw- Sat"(w140) -> ()
        n159 = local write "Sat-Log"(w144) -> ()
        n160 = local write "Raw- Lin"(w143) -> ()
        n161 = local write "Sqrt-Sat"(w139) -> ()
        n162 = local write "Log-Lin"(w141) -> ()
        n163 = local write "Sqrt-Lin"(w142) -> ()
      }
      frame "Re-Calculated Values" {
        n164 = local read "Vg Array-Log-Used"() -> (w197:dbl[])
        n165 = local read "Sat Vg Array-Used"() -> (w205:dbl[])
        n166 = local read "Lin-Vg Array-Used"() -> (w211:dbl[])
        n167 = local read "Sat Id-Log-Used"() -> (w196:dbl[])
        n168 = local read "New: Dielectric"() -> (w209:dbl)
        n169 = local read "New: Dielectric"() -> (w194:dbl)
        n170 = local read "New: Length"() -> (w208:dbl)
        n171 = local read "New: Length"() -> (w204:dbl)
        n172 = local read "New: Width"() -> (w207:dbl)
        n173 = local read "New: Width"() -> (w203:dbl)
        n174 = local read "Lin Id-Used"() -> (w210:dbl[])
        n175 = local read "Sat Id-Used"() -> (w202:dbl[])
        n176 = local read "Re-Calculated Values Cluster"() -> (w213:T9)
        n177 = local read "New: Dielectric"() -> (w193:dbl)
        n178 = local read "New: Temp"() -> (w192:dbl)
        n179 = local read "Lin Vd"() -> (w189:dbl)
        n180 = call "Mobility-Vt-Used Pts_Saturation.vi"("Width"=w203, "Length"=w204, "Dielectric (d)"=w194, "Sat Id Used"=w202, "Vg Used"=w205) -> ("Vt"=w200:dbl, "Mobility"=w201:dbl)  [unwired: 4 in, 1 out]
        n181 = call "STS-Used.vi"("Id Used"=w196, "Vg-Used"=w197) -> ("STS"=w195:dbl)  [unwired: 9 in]
        n182 = call "Mobility-Vt-Used Pts_Linear.vi"("Width"=w207, "Length"=w208, "Vd"=w189, "Dielectric (d)"=w209, "Id Used"=w210, "Vg Used"=w211) -> ("Mobility"=w206:dbl)  [unwired: 3 in, 2 out]
        n183 = call "Trap Density_VT.vi"("VT"=w200, "Dielectric"=w194) -> ("Trap Density-VT"=w199:dbl)
        n184 = call "Trap Density_STS.vi"("Temp (T) [K]"=w192, "S.T.S. (S)"=w195, "Dielectric"=w193) -> ("Trap Density (N)"=w191:dbl)  [unwired: 8 in]
        n185 = Bundle By Name(cluster=w213, "Mobility-Sat"=w201, "Moblitity-Lin"=w206, "Vt-Sat"=w200, "STS"=w195, "Trap Density-VT"=w199, "Trap Density-STS"=w191) -> (w212:T9)
        n186 = local write "Re-Calculated Values Cluster"(w212) -> ()
      }
      frame "Next File" {
        n187 = Strip Path(path=w230) -> (stripped path=w220:path, name=w228:string)
        n188 = local write "Transfer Folder"(w220) -> ()
        n189 = List Folder(path=w220) -> (filenames=w214:string[], error out=w223:errorcluster)  [unwired: 3 in, 2 out]
        n190 = Array Size(array=w214) -> (size(s)=w227:i32)
        n191 = Search 1D Array(1D array=w214, element=w228) -> (index of element=w225:i32)  [unwired: 1 in]
        n192 = Decrement(x=w227) -> (x-1=w226:i32)
        n193 = Equal?(x=w226, y=w225) -> (x = y?=w224:bool)
        n194 = case shown="False" w224 {
          tunnel: w216 -> [w233 _]
          tunnel: [w232 0] -> w215
          tunnel: w223 -> [w231 w234]
          tunnel: [w231 w234] -> _
          frame False {
            n195 = Increment(x=w233) -> (x+1=w232:i32)
          }
          frame True {
          }
        }
        n196 = Path To String(path=w220) -> (string=w221:string)
        n197 = Index Array(array=w214, index=w215) -> (element=w222:string)
        n198 = Concatenate Strings(w221, "\\", w222) -> (w218:string)
        n199 = String To Path(string=w218) -> (path=w217:path)
        n200 = local write "Transfer File"(w217) -> ()
      }
      frame "Previous File" {
        n201 = Strip Path(path=w242) -> (stripped path=w239:path, name=w251:string)
        n202 = local write "Transfer Folder"(w239) -> ()
        n203 = List Folder(path=w239) -> (filenames=w243:string[], error out=w248:errorcluster)  [unwired: 3 in, 2 out]
        n204 = Array Size(array=w243) -> (size(s)=w237:i32)
        n205 = Search 1D Array(1D array=w243, element=w251) -> (index of element=w250:i32)  [unwired: 1 in]
        n206 = Decrement(x=w237) -> (x-1=w236:i32)
        n207 = Equal To 0?(x=w250) -> (x = 0?=w249:bool)
        n208 = case shown="False" w249 {
          tunnel: w241 -> [w255 _]
          tunnel: [w254 w256] -> w240
          tunnel: w248 -> [w253 w257]
          tunnel: [w253 w257] -> _
          tunnel: w236 -> [_ w256]
          frame False {
            n209 = Decrement(x=w255) -> (x-1=w254:i32)
          }
          frame True {
          }
        }
        n210 = Path To String(path=w239) -> (string=w238:string)
        n211 = Index Array(array=w243, index=w240) -> (element=w247:string)
        n212 = Concatenate Strings(w238, "\\", w247) -> (w245:string)
        n213 = String To Path(string=w245) -> (path=w244:path)
        n214 = local write "Transfer File"(w244) -> ()
      }
      frame "Discard File" {
      }
      frame "Save" {
        n215 = stacked-sequence {
          seq-local: [w275 _] -> [_ w772]
          seq-local: [w274 _] -> [_ w770]
          tunnel: w266 -> [w276 w773]
          frame #0 {
            # "Saves each Re-calculated parameter in sequence"
            n216 = stacked-sequence {
              tunnel: [_ _ _ _ _ _ _ _ _ _ _ _ _ w740] -> w274
              tunnel: w276 -> [w296 _ _ _ _ _ _ _ _ _ _ _ _ _]
              frame #0 {
                n217 = call-poly <vilib>:"Read From Spreadsheet File.vi"("file path (dialog if empty)"=w296) -> ("all rows"=w295:string[][])  [unwired: 6 in, 4 out]
                n218 = Array Size(array=w295) -> (size(s)=w300:i32[])
                n219 = Array Subset(array=w295, index (row)=0, index (col)=0, length (col)=3) -> (w304:string[][])  [unwired: 1 in]
                n220 = Index Array(array=w300, index=0) -> (element=w298:i32)
                n221 = Reshape Array(w304, w298) -> (w297:string[])
                n222 = Search 1D Array(1D array=w297, element="Dielectric (nm):") -> (index of element=w307:i32)  [unwired: 1 in]
                n223 = Equal?(x=w307, y=-1) -> (x = y?=w306:bool)
                n224 = case shown="False" w306 {
                  tunnel: w295 -> [w315 w319]
                  tunnel: w307 -> [w311 _]
                  tunnel: [w310 w319] -> w305
                  frame False {
                    n225 = local read "Rec: Dielectric (d)"() -> (w317:dbl)
                    n226 = Number To Fractional String(number=w317) -> (F-format string=w312:string)  [unwired: 3 in]
                    n227 = Divide(x=w311, y=3) -> (x/y=w314:dbl)
                    n228 = To Word Integer(number=w314) -> (16bit integer=w313:i16)
                    n229 = Replace Array Subset(array=w315, new element=w312, index (row)=w313, index (col)=1) -> (w310:string[][])
                  }
                  frame True {
                  }
                }
                n230 = local write "Save Array"(w305) -> ()
              }
              frame #1 {
                n231 = local read "Save Array"() -> (w321:string[][])
                n232 = Array Size(array=w321) -> (size(s)=w324:i32[])
                n233 = Array Subset(array=w321, index (row)=0, index (col)=0, length (col)=3) -> (w328:string[][])  [unwired: 1 in]
                n234 = Index Array(array=w324, index=0) -> (element=w322:i32)
                n235 = Reshape Array(w328, w322) -> (w320:string[])
                n236 = Search 1D Array(1D array=w320, element="Comments:") -> (index of element=w331:i32)  [unwired: 1 in]
                n237 = Equal?(x=w331, y=-1) -> (x = y?=w330:bool)
                n238 = case shown="False" w330 {
                  tunnel: w321 -> [w339 w342]
                  tunnel: w331 -> [w336 _]
                  tunnel: [w335 w342] -> w329
                  frame False {
                    n239 = local read "New: Comments"() -> (w334:string)
                    n240 = Divide(x=w336, y=3) -> (x/y=w338:dbl)
                    n241 = To Word Integer(number=w338) -> (16bit integer=w337:i16)
                    n242 = Replace Array Subset(array=w339, new element=w334, index (row)=w337, index (col)=1) -> (w335:string[][])
                  }
                  frame True {
                  }
                }
                n243 = local write "Save Array"(w329) -> ()
              }
              frame #2 {
                n244 = local read "Save Array"() -> (w344:string[][])
                n245 = Array Size(array=w344) -> (size(s)=w347:i32[])
                n246 = Array Subset(array=w344, index (row)=0, index (col)=0, length (col)=3) -> (w351:string[][])  [unwired: 1 in]
                n247 = Index Array(array=w347, index=0) -> (element=w345:i32)
                n248 = Reshape Array(w351, w345) -> (w343:string[])
                n249 = Search 1D Array(1D array=w343, element="Length (um):") -> (index of element=w354:i32)  [unwired: 1 in]
                n250 = Equal?(x=w354, y=-1) -> (x = y?=w353:bool)
                n251 = case shown="False" w353 {
                  tunnel: w344 -> [w364 w367]
                  tunnel: w354 -> [w361 _]
                  tunnel: [w360 w367] -> w352
                  frame False {
                    n252 = local read "New: Length"() -> (w357:dbl)
                    n253 = Divide(x=w361, y=3) -> (x/y=w363:dbl)
                    n254 = Format Value(format string="%#g", value (0)=w357) -> (output string=w358:string)  [unwired: 1 in]
                    n255 = To Word Integer(number=w363) -> (16bit integer=w362:i16)
                    n256 = Replace Array Subset(array=w364, new element=w358, index (row)=w362, index (col)=1) -> (w360:string[][])
                  }
                  frame True {
                  }
                }
                n257 = local write "Save Array"(w352) -> ()
              }
              frame #3 {
                n258 = local read "Save Array"() -> (w369:string[][])
                n259 = Array Size(array=w369) -> (size(s)=w374:i32[])
                n260 = Array Subset(array=w369, index (row)=0, index (col)=0, length (col)=3) -> (w370:string[][])  [unwired: 1 in]
                n261 = Index Array(array=w374, index=0) -> (element=w376:i32)
                n262 = Reshape Array(w370, w376) -> (w368:string[])
                n263 = Search 1D Array(1D array=w368, element="Width (um):") -> (index of element=w379:i32)  [unwired: 1 in]
                n264 = Equal?(x=w379, y=-1) -> (x = y?=w378:bool)
                n265 = case shown="False" w378 {
                  tunnel: w379 -> [w387 _]
                  tunnel: w369 -> [w386 w392]
                  tunnel: [w385 w392] -> w377
                  frame False {
                    n266 = local read "New: Width"() -> (w382:dbl)
                    n267 = Divide(x=w387, y=3) -> (x/y=w389:dbl)
                    n268 = To Word Integer(number=w389) -> (16bit integer=w388:i16)
                    n269 = Format Value(format string="%#g", value (0)=w382) -> (output string=w383:string)  [unwired: 1 in]
                    n270 = Replace Array Subset(array=w386, new element=w383, index (row)=w388, index (col)=1) -> (w385:string[][])
                  }
                  frame True {
                  }
                }
                n271 = local write "Save Array"(w377) -> ()
              }
              frame #4 {
                w402 = "Sample Temp (K):"
                n272 = local read "Save Array"() -> (w394:string[][])
                n273 = Array Size(array=w394) -> (size(s)=w399:i32[])
                n274 = Array Subset(array=w394, index (row)=0, index (col)=0, length (col)=3) -> (w395:string[][])  [unwired: 1 in]
                n275 = Index Array(array=w399, index=0) -> (element=w401:i32)
                n276 = Reshape Array(w395, w401) -> (w393:string[])
                n277 = Search 1D Array(1D array=w393, element=w402) -> (index of element=w405:i32)  [unwired: 1 in]
                n278 = Equal?(x=w405, y=-1) -> (x = y?=w404:bool)
                n279 = case shown="False" w404 {
                  tunnel: w394 -> [w414 w428]
                  tunnel: w405 -> [w411 _]
                  tunnel: [w410 w427] -> w403
                  tunnel: w393 -> [_ w430]
                  tunnel: w402 -> [_ w417]
                  frame False {
                    n280 = local read "New: Temp"() -> (w408:dbl)
                    n281 = Divide(x=w411, y=3) -> (x/y=w413:dbl)
                    n282 = Format Value(format string="%#g", value (0)=w408) -> (output string=w407:string)  [unwired: 1 in]
                    n283 = To Word Integer(number=w413) -> (16bit integer=w412:i16)
                    n284 = Replace Array Subset(array=w414, new element=w407, index (row)=w412, index (col)=1) -> (w410:string[][])
                  }
                  frame True {
                    n285 = local read "New: Temp"() -> (w419:dbl)
                    n286 = Search 1D Array(1D array=w430, element="Width (um):") -> (index of element=w424:i32)  [unwired: 1 in]
                    n287 = Divide(x=w424, y=3) -> (x/y=w425:dbl)
                    n288 = To Word Integer(number=w425) -> (16bit integer=w423:i16)
                    n289 = Format Value(format string="%#g", value (0)=w419) -> (output string=w418:string)  [unwired: 1 in]
                    n290 = Build Array(w417, w418) -> (w421:string[])
                    n291 = Increment(x=w423) -> (x+1=w422:i16)
                    n292 = Insert Into Array(array=w428, index (row)=w422, new element=w421) -> (w427:string[][])  [unwired: 1 in]
                  }
                }
                n293 = local write "Save Array"(w403) -> ()
              }
              frame #5 {
                w440 = "Mobility-Sat (cm^2/Vs):"
                n294 = local read "Save Array"() -> (w432:string[][])
                n295 = Array Size(array=w432) -> (size(s)=w437:i32[])
                n296 = Array Subset(array=w432, index (row)=0, index (col)=0, length (col)=3) -> (w433:string[][])  [unwired: 1 in]
                n297 = Index Array(array=w437, index=0) -> (element=w439:i32)
                n298 = Reshape Array(w433, w439) -> (w431:string[])
                n299 = Search 1D Array(1D array=w431, element=w440) -> (index of element=w443:i32)  [unwired: 1 in]
                n300 = Equal?(x=w443, y=-1) -> (x = y?=w442:bool)
                n301 = case shown="False" w442 {
                  tunnel: w432 -> [w453 w463]
                  tunnel: w443 -> [w450 _]
                  tunnel: [w449 w462] -> w441
                  tunnel: w431 -> [_ w460]
                  tunnel: w440 -> [_ w458]
                  frame False {
                    n302 = local read "Re-Calculated Values Cluster"() -> (w446:T9)
                    n303 = Unbundle By Name(w446) -> ("Mobility-Sat"=w445:dbl)
                    n304 = Divide(x=w450, y=3) -> (x/y=w452:dbl)
                    n305 = To Word Integer(number=w452) -> (16bit integer=w451:i16)
                    n306 = Format Value(format string="%#g", value (0)=w445) -> (output string=w447:string)  [unwired: 1 in]
                    n307 = Replace Array Subset(array=w453, new element=w447, index (row)=w451, index (col)=1) -> (w449:string[][])
                  }
                  frame True {
                    n308 = local read "Re-Calculated Values Cluster"() -> (w457:T9)
                    n309 = Unbundle By Name(w457) -> ("Mobility-Sat"=w456:dbl)
                    n310 = Search 1D Array(1D array=w460, element="Mobility (cm^2/Vs):") -> (index of element=w466:i32)  [unwired: 1 in]
                    n311 = Divide(x=w466, y=3) -> (x/y=w467:dbl)
                    n312 = To Word Integer(number=w467) -> (16bit integer=w459:i16)
                    n313 = Format Value(format string="%#g", value (0)=w456) -> (output string=w461:string)  [unwired: 1 in]
                    n314 = Build Array(w458, w461) -> (w465:string[])
                    n315 = Replace Array Subset(array=w463, new element=w465, index (row)=w459) -> (w462:string[][])  [unwired: 1 in]
                  }
                }
                n316 = local write "Save Array"(w441) -> ()
              }
              frame #6 {
                w479 = "Mobility-Lin (cm^2/Vs):"
                n317 = local read "Save Array"() -> (w470:string[][])
                n318 = Array Size(array=w470) -> (size(s)=w476:i32[])
                n319 = Array Subset(array=w470, index (row)=0, index (col)=0, length (col)=3) -> (w472:string[][])  [unwired: 1 in]
                n320 = Index Array(array=w476, index=0) -> (element=w478:i32)
                n321 = Reshape Array(w472, w478) -> (w471:string[])
                n322 = Search 1D Array(1D array=w471, element=w479) -> (index of element=w482:i32)  [unwired: 1 in]
                n323 = Equal?(x=w482, y=-1) -> (x = y?=w481:bool)
                n324 = case shown="True" w481 {
                  tunnel: w470 -> [w492 w500]
                  tunnel: w482 -> [w489 _]
                  tunnel: [w488 w499] -> w480
                  tunnel: w471 -> [_ w498]
                  tunnel: w479 -> [_ w497]
                  frame False {
                    n325 = local read "Re-Calculated Values Cluster"() -> (w485:T9)
                    n326 = Unbundle By Name(w485) -> ("Moblitity-Lin"=w484:dbl)
                    n327 = Divide(x=w489, y=3) -> (x/y=w491:dbl)
                    n328 = To Word Integer(number=w491) -> (16bit integer=w490:i16)
                    n329 = Format Value(format string="%#g", value (0)=w484) -> (output string=w486:string)  [unwired: 1 in]
                    n330 = Replace Array Subset(array=w492, new element=w486, index (row)=w490, index (col)=1) -> (w488:string[][])
                  }
                  frame True {
                    n331 = local read "Re-Calculated Values Cluster"() -> (w496:T9)
                    n332 = Unbundle By Name(w496) -> ("Moblitity-Lin"=w495:dbl)
                    n333 = Search 1D Array(1D array=w498, element="Mobility-Sat (cm^2/Vs):") -> (index of element=w505:i32)  [unwired: 1 in]
                    n334 = Divide(x=w505, y=3) -> (x/y=w506:dbl)
                    n335 = To Word Integer(number=w506) -> (16bit integer=w504:i16)
                    n336 = Format Value(format string="%#g", value (0)=w495) -> (output string=w509:string)  [unwired: 1 in]
                    n337 = Build Array(w497, w509) -> (w502:string[])
                    n338 = Increment(x=w504) -> (x+1=w503:i16)
                    n339 = Insert Into Array(array=w500, index (row)=w503, new element=w502) -> (w499:string[][])  [unwired: 1 in]
                  }
                }
                n340 = local write "Save Array"(w480) -> ()
              }
              frame #7 {
                w519 = "On/Off I-Sat:"
                n341 = local read "Save Array"() -> (w510:string[][])
                n342 = Array Size(array=w510) -> (size(s)=w516:i32[])
                n343 = Array Subset(array=w510, index (row)=0, index (col)=0, length (col)=3) -> (w512:string[][])  [unwired: 1 in]
                n344 = Index Array(array=w516, index=0) -> (element=w518:i32)
                n345 = Reshape Array(w512, w518) -> (w511:string[])
                n346 = Search 1D Array(1D array=w511, element=w519) -> (index of element=w522:i32)  [unwired: 1 in]
                n347 = Equal?(x=w522, y=-1) -> (x = y?=w521:bool)
                n348 = case shown="True" w521 {
                  tunnel: w510 -> [w532 w541]
                  tunnel: w522 -> [w529 _]
                  tunnel: [w528 w542] -> w520
                  tunnel: w511 -> [_ w539]
                  tunnel: w519 -> [_ w537]
                  frame False {
                    n349 = local read "Re-Calculated Values Cluster"() -> (w525:T9)
                    n350 = Divide(x=w529, y=3) -> (x/y=w531:dbl)
                    n351 = Unbundle By Name(w525) -> ("On/Off"=w524:dbl)
                    n352 = To Word Integer(number=w531) -> (16bit integer=w530:i16)
                    n353 = Format Value(format string="%#g", value (0)=w524) -> (output string=w526:string)  [unwired: 1 in]
                    n354 = Replace Array Subset(array=w532, new element=w526, index (row)=w530, index (col)=1) -> (w528:string[][])
                  }
                  frame True {
                    n355 = local read "Re-Calculated Values Cluster"() -> (w536:T9)
                    n356 = Unbundle By Name(w536) -> ("On/Off"=w535:dbl)
                    n357 = Search 1D Array(1D array=w539, element="On/Off Current:") -> (index of element=w545:i32)  [unwired: 1 in]
                    n358 = Divide(x=w545, y=3) -> (x/y=w546:dbl)
                    n359 = To Word Integer(number=w546) -> (16bit integer=w538:i16)
                    n360 = Format Value(format string="%#g", value (0)=w535) -> (output string=w540:string)  [unwired: 1 in]
                    n361 = Build Array(w537, w540) -> (w544:string[])
                    n362 = Replace Array Subset(array=w541, new element=w544, index (row)=w538) -> (w542:string[][])  [unwired: 1 in]
                  }
                }
                n363 = local write "Save Array"(w520) -> ()
              }
              frame #8 {
                w558 = "Off I-Sat (A):"
                n364 = local read "Save Array"() -> (w549:string[][])
                n365 = Array Size(array=w549) -> (size(s)=w555:i32[])
                n366 = Array Subset(array=w549, index (row)=0, index (col)=0, length (col)=3) -> (w551:string[][])  [unwired: 1 in]
                n367 = Index Array(array=w555, index=0) -> (element=w557:i32)
                n368 = Reshape Array(w551, w557) -> (w550:string[])
                n369 = Search 1D Array(1D array=w550, element=w558) -> (index of element=w561:i32)  [unwired: 1 in]
                n370 = Equal?(x=w561, y=-1) -> (x = y?=w560:bool)
                n371 = case shown="True" w560 {
                  tunnel: w549 -> [w571 w579]
                  tunnel: w561 -> [w568 _]
                  tunnel: [w567 w578] -> w559
                  tunnel: w550 -> [_ w577]
                  tunnel: w558 -> [_ w576]
                  frame False {
                    n372 = local read "Re-Calculated Values Cluster"() -> (w564:T9)
                    n373 = Unbundle By Name(w564) -> ("Off Current"=w563:dbl)
                    n374 = Divide(x=w568, y=3) -> (x/y=w570:dbl)
                    n375 = Format Value(format string="%#g", value (0)=w563) -> (output string=w565:string)  [unwired: 1 in]
                    n376 = To Word Integer(number=w570) -> (16bit integer=w569:i16)
                    n377 = Replace Array Subset(array=w571, new element=w565, index (row)=w569, index (col)=1) -> (w567:string[][])
                  }
                  frame True {
                    n378 = local read "Re-Calculated Values Cluster"() -> (w575:T9)
                    n379 = Unbundle By Name(w575) -> ("Off Current"=w574:dbl)
                    n380 = Search 1D Array(1D array=w577, element="On/Off I-Sat:") -> (index of element=w584:i32)  [unwired: 1 in]
                    n381 = Divide(x=w584, y=3) -> (x/y=w585:dbl)
                    n382 = To Word Integer(number=w585) -> (16bit integer=w583:i16)
                    n383 = Format Value(format string="%#g", value (0)=w574) -> (output string=w588:string)  [unwired: 1 in]
                    n384 = Build Array(w576, w588) -> (w581:string[])
                    n385 = Increment(x=w583) -> (x+1=w582:i16)
                    n386 = Insert Into Array(array=w579, index (row)=w582, new element=w581) -> (w578:string[][])  [unwired: 1 in]
                  }
                }
                n387 = local write "Save Array"(w559) -> ()
              }
              frame #9 {
                w590 = "Vt-Sat (V):"
                n388 = local read "Save Array"() -> (w591:string[][])
                n389 = Array Size(array=w591) -> (size(s)=w596:i32[])
                n390 = Array Subset(array=w591, index (row)=0, index (col)=0, length (col)=3) -> (w592:string[][])  [unwired: 1 in]
                n391 = Index Array(array=w596, index=0) -> (element=w598:i32)
                n392 = Reshape Array(w592, w598) -> (w589:string[])
                n393 = Search 1D Array(1D array=w589, element=w590) -> (index of element=w601:i32)  [unwired: 1 in]
                n394 = Equal?(x=w601, y=-1) -> (x = y?=w600:bool)
                n395 = case shown="False" w600 {
                  tunnel: w591 -> [w610 w620]
                  tunnel: w601 -> [w606 _]
                  tunnel: [w605 w619] -> w599
                  tunnel: w590 -> [_ w618]
                  tunnel: w589 -> [_ w617]
                  frame False {
                    n396 = local read "Re-Calculated Values Cluster"() -> (w604:T9)
                    n397 = Unbundle By Name(w604) -> ("Vt-Sat"=w603:dbl)
                    n398 = Divide(x=w606, y=3) -> (x/y=w609:dbl)
                    n399 = To Word Integer(number=w609) -> (16bit integer=w608:i16)
                    n400 = Number To Fractional String(number=w603) -> (F-format string=w607:string)  [unwired: 3 in]
                    n401 = Replace Array Subset(array=w610, new element=w607, index (row)=w608, index (col)=1) -> (w605:string[][])
                  }
                  frame True {
                    n402 = local read "Re-Calculated Values Cluster"() -> (w614:T9)
                    n403 = Unbundle By Name(w614) -> ("Vt-Sat"=w613:dbl)
                    n404 = Search 1D Array(1D array=w617, element="Threshold V (V):") -> (index of element=w616:i32)  [unwired: 1 in]
                    n405 = Divide(x=w616, y=3) -> (x/y=w623:dbl)
                    n406 = To Word Integer(number=w623) -> (16bit integer=w615:i16)
                    n407 = Format Value(format string="%#g", value (0)=w613) -> (output string=w626:string)  [unwired: 1 in]
                    n408 = Build Array(w618, w626) -> (w622:string[])
                    n409 = Replace Array Subset(array=w620, new element=w622, index (row)=w615) -> (w619:string[][])  [unwired: 1 in]
                  }
                }
                n410 = local write "Save Array"(w599) -> ()
              }
              frame #10 {
                n411 = disable-structure shown="Disabled" {
                  frame Disabled {
                    n412 = local read "Save Array"() -> (w627:string[][])
                    n413 = Array Size(array=w627) -> (size(s)=w633:i32[])
                    n414 = Array Subset(array=w627, index (row)=0, index (col)=0, length (col)=3) -> (w629:string[][])  [unwired: 1 in]
                    n415 = Index Array(array=w633, index=0) -> (element=w635:i32)
                    n416 = Reshape Array(w629, w635) -> (w628:string[])
                    n417 = Search 1D Array(1D array=w628, element="VT-Lin (V):") -> (index of element=w638:i32)  [unwired: 1 in]
                    n418 = Equal?(x=w638, y=-1) -> (x = y?=w637:bool)
                    n419 = case shown="False" w637 {
                      tunnel: w627 -> [w647 w650]
                      tunnel: w638 -> [w644 _]
                      tunnel: [w643 w650] -> w636
                      frame False {
                        n420 = Divide(x=w644, y=3) -> (x/y=w646:dbl)
                        n421 = To Word Integer(number=w646) -> (16bit integer=w645:i16)
                        n422 = Format Value(format string="%#g") -> (output string=w641:string)  [unwired: 2 in]
                        n423 = Replace Array Subset(array=w647, new element=w641, index (row)=w645, index (col)=1) -> (w643:string[][])
                      }
                      frame True {
                      }
                    }
                    n424 = local write "Save Array"(w636) -> ()
                  }
                  frame Enabled {
                  }
                }
              }
              frame #11 {
                w651 = "STS-Sat (V/decade):"
                n425 = local read "Save Array"() -> (w653:string[][])
                n426 = Array Size(array=w653) -> (size(s)=w658:i32[])
                n427 = Array Subset(array=w653, index (row)=0, index (col)=0, length (col)=3) -> (w654:string[][])  [unwired: 1 in]
                n428 = Index Array(array=w658, index=0) -> (element=w660:i32)
                n429 = Reshape Array(w654, w660) -> (w652:string[])
                n430 = Search 1D Array(1D array=w652, element=w651) -> (index of element=w663:i32)  [unwired: 1 in]
                n431 = Equal?(x=w663, y=-1) -> (x = y?=w662:bool)
                n432 = case shown="True" w662 {
                  tunnel: w653 -> [w673 w681]
                  tunnel: w663 -> [w670 _]
                  tunnel: [w669 w682] -> w661
                  tunnel: w652 -> [_ w680]
                  tunnel: w651 -> [_ w679]
                  frame False {
                    n433 = local read "Re-Calculated Values Cluster"() -> (w665:T9)
                    n434 = Unbundle By Name(w665) -> ("STS"=w666:dbl)
                    n435 = Divide(x=w670, y=3) -> (x/y=w672:dbl)
                    n436 = To Word Integer(number=w672) -> (16bit integer=w671:i16)
                    n437 = Format Value(format string="%#g", value (0)=w666) -> (output string=w667:string)  [unwired: 1 in]
                    n438 = Replace Array Subset(array=w673, new element=w667, index (row)=w671, index (col)=1) -> (w669:string[][])
                  }
                  frame True {
                    n439 = local read "Re-Calculated Values Cluster"() -> (w676:T9)
                    n440 = Unbundle By Name(w676) -> ("STS"=w677:dbl)
                    n441 = Search 1D Array(1D array=w680, element="S.T.S. (V/decade):") -> (index of element=w685:i32)  [unwired: 1 in]
                    n442 = Divide(x=w685, y=3) -> (x/y=w686:dbl)
                    n443 = To Word Integer(number=w686) -> (16bit integer=w678:i16)
                    n444 = Format Value(format string="%#g", value (0)=w677) -> (output string=w689:string)  [unwired: 1 in]
                    n445 = Build Array(w679, w689) -> (w684:string[])
                    n446 = Replace Array Subset(array=w681, new element=w684, index (row)=w678) -> (w682:string[][])  [unwired: 1 in]
                  }
                }
                n447 = local write "Save Array"(w661) -> ()
              }
              frame #12 {
                w690 = "Trap Density-VT (Traps/Vcm^2):"
                n448 = local read "Save Array"() -> (w692:string[][])
                n449 = Array Size(array=w692) -> (size(s)=w697:i32[])
                n450 = Array Subset(array=w692, index (row)=0, index (col)=0, length (col)=3) -> (w693:string[][])  [unwired: 1 in]
                n451 = Index Array(array=w697, index=0) -> (element=w699:i32)
                n452 = Reshape Array(w693, w699) -> (w691:string[])
                n453 = Search 1D Array(1D array=w691, element=w690) -> (index of element=w702:i32)  [unwired: 1 in]
                n454 = Equal?(x=w702, y=-1) -> (x = y?=w701:bool)
                n455 = case shown="True" w701 {
                  tunnel: w692 -> [w712 w719]
                  tunnel: w702 -> [w708 _]
                  tunnel: [w707 w720] -> w700
                  tunnel: w691 -> [_ w718]
                  tunnel: w690 -> [_ w717]
                  frame False {
                    n456 = local read "Re-Calculated Values Cluster"() -> (w705:T9)
                    n457 = Unbundle By Name(w705) -> ("Trap Density-VT"=w704:dbl)
                    n458 = Divide(x=w708, y=3) -> (x/y=w711:dbl)
                    n459 = To Word Integer(number=w711) -> (16bit integer=w710:i16)
                    n460 = Format Value(format string="%#g", value (0)=w704) -> (output string=w709:string)  [unwired: 1 in]
                    n461 = Replace Array Subset(array=w712, new element=w709, index (row)=w710, index (col)=1) -> (w707:string[][])
                  }
                  frame True {
                    n462 = local read "Re-Calculated Values Cluster"() -> (w716:T9)
                    n463 = Unbundle By Name(w716) -> ("Trap Density-VT"=w715:dbl)
                    n464 = Search 1D Array(1D array=w718, element="STS-Sat (V/decade):") -> (index of element=w725:i32)  [unwired: 1 in]
                    n465 = Divide(x=w725, y=3) -> (x/y=w724:dbl)
                    n466 = To Word Integer(number=w724) -> (16bit integer=w726:i16)
                    n467 = Format Value(format string="%#g", value (0)=w715) -> (output string=w721:string)  [unwired: 1 in]
                    n468 = Build Array(w717, w721) -> (w728:string[])
                    n469 = Increment(x=w726) -> (x+1=w727:i16)
                    n470 = Insert Into Array(array=w719, index (row)=w727, new element=w728) -> (w720:string[][])  [unwired: 1 in]
                  }
                }
                n471 = local write "Save Array"(w700) -> ()
              }
              frame #13 {
                w730 = "Trap Density-STS (Traps/Vcm^2):"
                n472 = local read "Save Array"() -> (w732:string[][])
                n473 = Array Size(array=w732) -> (size(s)=w737:i32[])
                n474 = Array Subset(array=w732, index (row)=0, index (col)=0, length (col)=3) -> (w733:string[][])  [unwired: 1 in]
                n475 = Index Array(array=w737, index=0) -> (element=w739:i32)
                n476 = Reshape Array(w733, w739) -> (w731:string[])
                n477 = Search 1D Array(1D array=w731, element=w730) -> (index of element=w742:i32)  [unwired: 1 in]
                n478 = Equal?(x=w742, y=-1) -> (x = y?=w741:bool)
                n479 = case shown="True" w741 {
                  tunnel: w732 -> [w752 w759]
                  tunnel: w742 -> [w749 _]
                  tunnel: [w748 w760] -> w740
                  tunnel: w731 -> [_ w758]
                  tunnel: w730 -> [_ w757]
                  frame False {
                    n480 = local read "Re-Calculated Values Cluster"() -> (w745:T9)
                    n481 = Unbundle By Name(w745) -> ("Trap Density-STS"=w744:dbl)
                    n482 = Divide(x=w749, y=3) -> (x/y=w751:dbl)
                    n483 = To Word Integer(number=w751) -> (16bit integer=w750:i16)
                    n484 = Format Value(format string="%#g", value (0)=w744) -> (output string=w746:string)  [unwired: 1 in]
                    n485 = Replace Array Subset(array=w752, new element=w746, index (row)=w750, index (col)=1) -> (w748:string[][])
                  }
                  frame True {
                    n486 = local read "Re-Calculated Values Cluster"() -> (w756:T9)
                    n487 = Unbundle By Name(w756) -> ("Trap Density-STS"=w755:dbl)
                    n488 = Search 1D Array(1D array=w758, element="Trap Density-VT (Traps/Vcm^2):") -> (index of element=w765:i32)  [unwired: 1 in]
                    n489 = Divide(x=w765, y=3) -> (x/y=w766:dbl)
                    n490 = To Word Integer(number=w766) -> (16bit integer=w764:i16)
                    n491 = Format Value(format string="%#g", value (0)=w755) -> (output string=w769:string)  [unwired: 1 in]
                    n492 = Build Array(w757, w769) -> (w762:string[])
                    n493 = Increment(x=w764) -> (x+1=w763:i16)
                    n494 = Insert Into Array(array=w759, index (row)=w763, new element=w762) -> (w760:string[][])  [unwired: 1 in]
                  }
                }
                n495 = local write "Save Array"(w740) -> ()
              }
            }
            n496 = local read "New: Temp"() -> (w277:dbl)
            n497 = local read "New: Width"() -> (w278:dbl)
            n498 = local read "New: Length"() -> (w280:dbl)
            n499 = local read "Index"() -> (w279:string)
            n500 = To Single Precision Float(number=w277) -> (single precision float=w294:sgl)
            n501 = Number To Decimal String(number=w294) -> (decimal integer string=w289:string)  [unwired: 1 in]
            n502 = To Single Precision Float(number=w278) -> (single precision float=w293:sgl)
            n503 = To Single Precision Float(number=w280) -> (single precision float=w292:sgl)
            n504 = Strip Path(path=w276) -> (stripped path=w281:path)  [unwired: 1 out]
            n505 = Number To Decimal String(number=w292) -> (decimal integer string=w287:string)  [unwired: 1 in]
            n506 = Number To Decimal String(number=w293) -> (decimal integer string=w286:string)  [unwired: 1 in]
            n507 = Concatenate Strings("_", w289, "K") -> (w291:string)
            n508 = call "Build Text"("Temp"=w291, "Index"=w279, "Length"=w287, "Width"=w286) -> ("Result"=w285:string)  [unwired: 10 in, 1 out]
            n509 = Path To String(path=w281) -> (string=w283:string)
            n510 = Concatenate Strings(w283, "\\", w285) -> (w284:string)
            n511 = String To Path(string=w284) -> (path=w275:path)
          }
          frame #1 {
            n512 = flat-sequence {
              tunnel: w773 -> [w775]
              tunnel: w772 -> [w774]
              tunnel: [w774] -> w771
              tunnel: w771 -> [w781]
              tunnel: w770 -> [w780]
              frame #0 {
                n513 = Equal?(x=w775, y=w774) -> (x = y?=w776:bool)
                n514 = case shown="False" w776 {
                  tunnel: w775 -> [w779 _]
                  tunnel: w774 -> [w778 _]
                  frame False {
                    n515 = Move(source path=w779, 9:TRUE, 10:w778) -> ()  [unwired: 2 in, 3 out]
                  }
                  frame True {
                  }
                }
              }
              frame #1 {
                n516 = local write "Transfer File"(w781) -> ()
                n517 = call-poly <vilib>:"Write To Spreadsheet File.vi"("2D data"=w780, "file path (dialog if empty)"=w781) -> ()  [unwired: 6 in, 1 out]
              }
            }
          }
        }
        n518 = Cluster To Array(cluster=w265) -> (array=w264:bool[])
        n519 = Boolean Array To Number(Boolean array=w264) -> (number=w263:u32)
        n520 = Equal To 0?(x=w263) -> (x = 0?=w262:bool)
        n521 = case shown="True" w262 {
          tunnel: [MegaAwesome_States."Read Data" w269] -> w261
          tunnel: w260 -> [_ w273]
          frame False {
          }
          frame True {
            n522 = Unbundle By Name(w273) -> ("Save Next"=w272:bool)
            n523 = Select(t=MegaAwesome_States."No Event", s=w272, f=MegaAwesome_States."Next File") -> (s? t:f=w269:T2)
          }
        }
      }
      frame "Exit" {
      }
      frame "Save Lines" {
      }
      frame "Export" {
        n524 = flat-sequence {
          frame #0 {
            n525 = stacked-sequence {
              frame #0 {
                n526 = local read "Independant Variable:"() -> (w788:string)
                n527 = Equal?(x=w788, y="Length (um):") -> (x = y?=w789:bool)
                n528 = case shown="True" w789 {
                  frame False {
                  }
                  frame True {
                    n529 = local write "X Axis Display Type"("1") -> ()
                    n530 = local write "Opj X Axis"("2") -> ()
                  }
                }
              }
              frame #1 {
                n531 = local read "Independant Variable:"() -> (w793:string)
                n532 = Equal?(x=w793, y="Sample Temp (K):") -> (x = y?=w794:bool)
                n533 = case shown="True" w794 {
                  frame False {
                  }
                  frame True {
                    n534 = local write "X Axis Display Type"("1") -> ()
                    n535 = local write "Opj X Axis"("1") -> ()
                  }
                }
              }
              frame #2 {
                n536 = local read "Independant Variable:"() -> (w798:string)
                n537 = Equal?(x=w798, y="Mobility-Sat (cm^2/Vs):") -> (x = y?=w799:bool)
                n538 = case shown="True" w799 {
                  frame False {
                  }
                  frame True {
                    n539 = local write "X Axis Display Type"("2") -> ()
                    n540 = local write "Opj X Axis"("2") -> ()
                  }
                }
              }
              frame #3 {
                n541 = local read "Independant Variable:"() -> (w803:string)
                n542 = Equal?(x=w803, y="Mobility-Lin (cm^2/Vs):") -> (x = y?=w804:bool)
                n543 = case shown="True" w804 {
                  frame False {
                  }
                  frame True {
                    n544 = local write "X Axis Display Type"("2") -> ()
                    n545 = local write "Opj X Axis"("2") -> ()
                  }
                }
              }
              frame #4 {
                n546 = local read "Independant Variable:"() -> (w808:string)
                n547 = Equal?(x=w808, y="On/Off I-Sat:") -> (x = y?=w809:bool)
                n548 = case shown="True" w809 {
                  frame False {
                  }
                  frame True {
                    n549 = local write "X Axis Display Type"("2") -> ()
                    n550 = local write "Opj X Axis"("2") -> ()
                  }
                }
              }
              frame #5 {
                n551 = local read "Independant Variable:"() -> (w813:string)
                n552 = Equal?(x=w813, y="Off I-Sat (A):") -> (x = y?=w814:bool)
                n553 = case shown="True" w814 {
                  frame False {
                  }
                  frame True {
                    n554 = local write "X Axis Display Type"("2") -> ()
                    n555 = local write "Opj X Axis"("2") -> ()
                  }
                }
              }
              frame #6 {
                n556 = local read "Independant Variable:"() -> (w818:string)
                n557 = Equal?(x=w818, y="Vt-Sat (V):") -> (x = y?=w819:bool)
                n558 = case shown="True" w819 {
                  frame False {
                  }
                  frame True {
                    n559 = local write "X Axis Display Type"("1") -> ()
                    n560 = local write "Opj X Axis"("1") -> ()
                  }
                }
              }
              frame #7 {
                n561 = local read "Independant Variable:"() -> (w823:string)
                n562 = Equal?(x=w823, y="STS-Sat (V/decade):") -> (x = y?=w824:bool)
                n563 = case shown="True" w824 {
                  frame False {
                  }
                  frame True {
                    n564 = local write "X Axis Display Type"("1") -> ()
                    n565 = local write "Opj X Axis"("1") -> ()
                  }
                }
              }
              frame #8 {
                n566 = local read "Independant Variable:"() -> (w828:string)
                n567 = Equal?(x=w828, y="Trap Density-VT (Traps/Vcm^2):") -> (x = y?=w829:bool)
                n568 = case shown="True" w829 {
                  frame False {
                  }
                  frame True {
                    n569 = local write "X Axis Display Type"("2") -> ()
                    n570 = local write "Opj X Axis"("2") -> ()
                  }
                }
              }
              frame #9 {
                n571 = local read "Independant Variable:"() -> (w833:string)
                n572 = Equal?(x=w833, y="Trap Density-STS (Traps/Vcm^2):") -> (x = y?=w834:bool)
                n573 = case shown="True" w834 {
                  frame False {
                  }
                  frame True {
                    n574 = local write "X Axis Display Type"("2") -> ()
                    n575 = local write "Opj X Axis"("2") -> ()
                  }
                }
              }
            }
          }
          frame #1 {
            n576 = local read "Transfer Folder"() -> (w842:path)
            n577 = Build Path(base path=w842, name or relative path="Stats") -> (appended path=w843:path)
            n578 = local read "Origin Project File"() -> (w854:path)
            n579 = call <vilib>:"Check if File or Folder Exists.vi"("path"=w843) -> ("file or folder exists?"=w858:bool, "dup path"=w857:path)  [unwired: 8 in, 1 out]
            n580 = call <userlib>:"OA_ConnectToOrigin.vi"() -> ("error out"=w855:errorcluster, "Origin.IOApplication"=w856:refnum<k7>)  [unwired: 8 in]
            n581 = case shown="False" w858 {
              tunnel: w857 -> [w1031 w1032]
              tunnel: [w1030 w1032] -> w841
              frame False {
                n582 = Create Folder(path (use dialog)=w1031) -> (created path=w1030:path)  [unwired: 2 in, 2 out]
              }
              frame True {
              }
            }
            n583 = call "File Dialog"("start path"=w843) -> ("selected path"=w845:path)  [unwired: 11 in, 3 out]
            n584 = call <userlib>:"OA_Load.vi"("error in (no error)"=w855, "Path"=w854, "Origin.IOApplication"=w856) -> ("error out"=w852:errorcluster, "Origin.IOApplication"=w853:refnum<k7>)  [unwired: 1 out]
            n585 = call "OAExecute.vi"("script"="document -m 3;", "Error IO"=w852, "Origin.IOApplication"=w853) -> ("Error IO Out"=w850:errorcluster, "Origin.IOApplication"=w851:refnum<k7>)  [unwired: 1 in, 1 out]
            n586 = local read "Independant Variable:"() -> (w838:string)
            n587 = stacked-sequence {
              tunnel: w842 -> [w869 w899 w911 w933 w953 w974 w995 w1018]
              tunnel: w841 -> [w870 w898 w912 w932 w954 w975 w996 w1019]
              tunnel: w851 -> [w872 w896 w914 w935 w956 w977 w998 w1021]
              tunnel: w850 -> [w871 w897 w913 w934 w955 w976 w997 w1020]
              tunnel: [_ _ _ _ _ _ _ w1016] -> w840
              tunnel: [_ _ _ _ _ _ _ w1017] -> w839
              tunnel: w838 -> [w868 w889 w910 w931 w952 w973 w994 w1015]
              frame #0 {
                n588 = local read "X Axis Display Type"() -> (w860:string)
                n589 = local read "Opj X Axis"() -> (w865:string)
                n590 = Concatenate Strings("window -a MOBLGraph;\nlayer.x.type=", w865, "; layer.x.label.numFormat = ", w860, "; Y3 = 1; X3 = 1;", "window -a MOBLTable;\nwindow -s TV;") -> (w863:string)
                n591 = call "Param_Analysis_7_24b_JW.vi"("Independant Variable"=w868, "error in (no error)"=w871, "Data Folder"=w869, "Parameter String"="Mobility-Lin (cm^2/Vs):", "Parameter Name"="Mobility-Lin", "Stats Folder"=w870) -> ("error out"=w874:errorcluster, "Output Array"=w876:string[][], "Variables"=w867:T15)  [unwired: 2 in, 1 out]
                n592 = call "Origin_Export_7_27a_JW.vi"("Input Conditions"=w867, "Analysis Array"=w876, "error in (no error)"=w874, "Parameter Worksheet Name"="[MOBLTable]Mobilities", "Parameter Folder Script"="pe_cd \"Mobility-Lin\";", "Origin.IOApplication"=w872) -> ("error out"=w873:errorcluster, "reference out"=w875:refnum<k7>)  [unwired: 3 in, 1 out]
                n593 = call "OAExecute.vi"("script"=w863, "Error IO"=w873, "Origin.IOApplication"=w875) -> ()  [unwired: 1 in, 3 out]
              }
              frame #1 {
                n594 = local read "X Axis Display Type"() -> (w881:string)
                n595 = local read "Opj X Axis"() -> (w886:string)
                n596 = Concatenate Strings("window -a MOBSGraph;\nlayer.x.type=", w886, "; layer.x.label.numFormat = ", w881, "; Y3 = 1; X3 = 1;", "window -a MOBSTable;\nwindow -s TV;") -> (w884:string)
                n597 = call "Param_Analysis_7_24b_JW.vi"("Independant Variable"=w889, "error in (no error)"=w897, "Data Folder"=w899, "Parameter String"="Mobility-Sat (cm^2/Vs):", "Parameter Name"="Mobility-Sat", "Stats Folder"=w898) -> ("error out"=w892:errorcluster, "Output Array"=w890:string[][], "Variables"=w888:T15)  [unwired: 2 in, 1 out]
                n598 = call "Origin_Export_7_27a_JW.vi"("Input Conditions"=w888, "Analysis Array"=w890, "error in (no error)"=w892, "Parameter Worksheet Name"="[MOBSTable]Mobilities", "Parameter Folder Script"="pe_cd \"Mobility-Sat\";", "Origin.IOApplication"=w896) -> ("error out"=w891:errorcluster, "reference out"=w893:refnum<k7>)  [unwired: 3 in, 1 out]
                n599 = call "OAExecute.vi"("script"=w884, "Error IO"=w891, "Origin.IOApplication"=w893) -> ()  [unwired: 1 in, 3 out]
              }
              frame #2 {
                n600 = local read "X Axis Display Type"() -> (w902:string)
                n601 = local read "Opj X Axis"() -> (w907:string)
                n602 = Concatenate Strings("window -a NSTSGraph;\nlayer.x.type=", w907, "; layer.x.label.numFormat = ", w902, "; Y3 = 1; X3 = 1;", "window -a NSTSTable;\nwindow -s TV;") -> (w905:string)
                n603 = call "Param_Analysis_7_24b_JW.vi"("Independant Variable"=w910, "error in (no error)"=w913, "Data Folder"=w911, "Parameter String"="Trap Density-STS (Traps/Vcm^2):", "Parameter Name"="Trap Density-STS", "Stats Folder"=w912) -> ("error out"=w917:errorcluster, "Output Array"=w915:string[][], "Variables"=w909:T15)  [unwired: 2 in, 1 out]
                n604 = call "Origin_Export_7_27a_JW.vi"("Input Conditions"=w909, "Analysis Array"=w915, "error in (no error)"=w917, "Parameter Worksheet Name"="[NSTSTable]Trap Densities", "Parameter Folder Script"="pe_cd \"N-STS\";", "Origin.IOApplication"=w914) -> ("error out"=w916:errorcluster, "reference out"=w918:refnum<k7>)  [unwired: 3 in, 1 out]
                n605 = call "OAExecute.vi"("script"=w905, "Error IO"=w916, "Origin.IOApplication"=w918) -> ()  [unwired: 1 in, 3 out]
              }
              frame #3 {
                n606 = local read "X Axis Display Type"() -> (w923:string)
                n607 = local read "Opj X Axis"() -> (w928:string)
                n608 = call "Param_Analysis_7_24b_JW.vi"("Independant Variable"=w931, "error in (no error)"=w934, "Data Folder"=w933, "Parameter String"="Trap Density-VT (Traps/Vcm^2):", "Parameter Name"="Trap Density-Vt", "Stats Folder"=w932) -> ("error out"=w938:errorcluster, "Output Array"=w936:string[][], "Variables"=w930:T15)  [unwired: 2 in, 1 out]
                n609 = Concatenate Strings("window -a NVtGraph;\nlayer.x.type=", w928, "; layer.x.label.numFormat = ", w923, "; Y3 = 1; X3 = 1;", "window -a NVtTable;\nwindow -s TV;") -> (w926:string)
                n610 = call "Origin_Export_7_27a_JW.vi"("Input Conditions"=w930, "Analysis Array"=w936, "error in (no error)"=w938, "Parameter Worksheet Name"="[NVTTable]Trap Densities", "Parameter Folder Script"="pe_cd \"N-Vt\";", "Origin.IOApplication"=w935) -> ("error out"=w937:errorcluster, "reference out"=w939:refnum<k7>)  [unwired: 3 in, 1 out]
                n611 = call "OAExecute.vi"("script"=w926, "Error IO"=w937, "Origin.IOApplication"=w939) -> ()  [unwired: 1 in, 3 out]
              }
              frame #4 {
                n612 = local read "X Axis Display Type"() -> (w944:string)
                n613 = local read "Opj X Axis"() -> (w949:string)
                n614 = Concatenate Strings("window -a OffIGraph;\nlayer.x.type=", w949, "; layer.x.label.numFormat = ", w944, "; Y3 = 1; X3 = 1;", "window -a OffITable;\nwindow -s TV;") -> (w947:string)
                n615 = call "Param_Analysis_7_24b_JW.vi"("Independant Variable"=w952, "error in (no error)"=w955, "Data Folder"=w953, "Parameter String"="Off I-Sat (A):", "Parameter Name"="Off I-Sat", "Stats Folder"=w954) -> ("error out"=w959:errorcluster, "Output Array"=w957:string[][], "Variables"=w951:T15)  [unwired: 2 in, 1 out]
                n616 = call "Origin_Export_7_27a_JW.vi"("Input Conditions"=w951, "Analysis Array"=w957, "error in (no error)"=w959, "Parameter Worksheet Name"="[OffItable]OffCurrents", "Parameter Folder Script"="pe_cd \"OffI-Sat\";", "Origin.IOApplication"=w956) -> ("error out"=w958:errorcluster, "reference out"=w960:refnum<k7>)  [unwired: 3 in, 1 out]
                n617 = call "OAExecute.vi"("script"=w947, "Error IO"=w958, "Origin.IOApplication"=w960) -> ()  [unwired: 1 in, 3 out]
              }
              frame #5 {
                n618 = local read "X Axis Display Type"() -> (w965:string)
                n619 = local read "Opj X Axis"() -> (w970:string)
                n620 = Concatenate Strings("window -a OnOffGraph;\nlayer.x.type=", w970, "; layer.x.label.numFormat = ", w965, "; Y3 = 1; X3 = 1;", "window -a OnOffTable;\nwindow -s TV;") -> (w968:string)
                n621 = call "Param_Analysis_7_24b_JW.vi"("Independant Variable"=w973, "error in (no error)"=w976, "Data Folder"=w974, "Parameter String"="On/Off I-Sat:", "Parameter Name"="OnOff Ratio", "Stats Folder"=w975) -> ("error out"=w980:errorcluster, "Output Array"=w978:string[][], "Variables"=w972:T15)  [unwired: 2 in, 1 out]
                n622 = call "Origin_Export_7_27a_JW.vi"("Input Conditions"=w972, "Analysis Array"=w978, "error in (no error)"=w980, "Parameter Worksheet Name"="[OnOffTable]On/Off Ratios", "Parameter Folder Script"="pe_cd \"OnOff-Ratio\";", "Origin.IOApplication"=w977) -> ("error out"=w979:errorcluster, "reference out"=w981:refnum<k7>)  [unwired: 3 in, 1 out]
                n623 = call "OAExecute.vi"("script"=w968, "Error IO"=w979, "Origin.IOApplication"=w981) -> ()  [unwired: 1 in, 3 out]
              }
              frame #6 {
                n624 = local read "X Axis Display Type"() -> (w986:string)
                n625 = local read "Opj X Axis"() -> (w991:string)
                n626 = call "Param_Analysis_7_24b_JW.vi"("Independant Variable"=w994, "error in (no error)"=w997, "Data Folder"=w995, "Parameter String"="STS-Sat (V/decade):", "Parameter Name"="STS-Sat", "Stats Folder"=w996) -> ("error out"=w1001:errorcluster, "Output Array"=w999:string[][], "Variables"=w993:T15)  [unwired: 2 in, 1 out]
                n627 = Concatenate Strings("window -a SGraph;\nlayer.x.type=", w991, "; layer.x.label.numFormat = ", w986, "; Y3 = 1; X3 = 1;", "window -a STable;\nwindow -s TV;") -> (w989:string)
                n628 = call "Origin_Export_7_27a_JW.vi"("Input Conditions"=w993, "Analysis Array"=w999, "error in (no error)"=w1001, "Parameter Worksheet Name"="[STable]Threshold Swing", "Parameter Folder Script"="pe_cd \"STS-Sat\";", "Origin.IOApplication"=w998) -> ("error out"=w1000:errorcluster, "reference out"=w1002:refnum<k7>)  [unwired: 3 in, 1 out]
                n629 = call "OAExecute.vi"("script"=w989, "Error IO"=w1000, "Origin.IOApplication"=w1002) -> ()  [unwired: 1 in, 3 out]
              }
              frame #7 {
                n630 = local read "X Axis Display Type"() -> (w1007:string)
                n631 = local read "Opj X Axis"() -> (w1012:string)
                n632 = Concatenate Strings("window -a VtGraph;\nlayer.x.type=", w1012, "; layer.x.label.numFormat = ", w1007, "; Y3 = 1; X3 = 1;", "window -a VtTable;\nwindow -s TV;") -> (w1010:string)
                n633 = call "Param_Analysis_7_24b_JW.vi"("Independant Variable"=w1015, "error in (no error)"=w1020, "Data Folder"=w1018, "Parameter String"="Vt-Sat (V):", "Parameter Name"="Vt-Sat", "Stats Folder"=w1019) -> ("error out"=w1024:errorcluster, "Output Array"=w1022:string[][], "Variables"=w1014:T15)  [unwired: 2 in, 1 out]
                n634 = call "Origin_Export_7_27a_JW.vi"("Input Conditions"=w1014, "Analysis Array"=w1022, "error in (no error)"=w1024, "Parameter Worksheet Name"="[VtTable]Threshold Voltages", "Parameter Folder Script"="pe_cd \"Vt-Sat\";", "Origin.IOApplication"=w1021) -> ("error out"=w1023:errorcluster, "reference out"=w1025:refnum<k7>)  [unwired: 3 in, 1 out]
                n635 = call "OAExecute.vi"("script"=w1010, "Error IO"=w1023, "Origin.IOApplication"=w1025) -> ("Error IO Out"=w1016:errorcluster, "Origin.IOApplication"=w1017:refnum<k7>)  [unwired: 1 in, 1 out]
              }
            }
            n636 = Path To String(path=w845) -> (string=w844:string)
            n637 = call "OAExecute.vi"("script"="pe_cd /; ", "Error IO"=w840, "Origin.IOApplication"=w839) -> ("Error IO Out"=w846:errorcluster, "Origin.IOApplication"=w847:refnum<k7>)  [unwired: 1 in, 1 out]
            n638 = call <userlib>:"OASaveProject.vi"("path"=w844, "Error IO"=w846, "Origin.IOApplication"=w847) -> ()  [unwired: 3 out]
          }
        }
      }
    }
    "Current State" <- w13
    "Folder Index" <- w6
    n639 = Equal?(x=w15, y=MegaAwesome_States."Exit") -> (x = y?=w16:bool)
    n640 = Wait (ms)(milliseconds to wait=5) -> ()  [unwired: 1 out]
  }
